vi "ATF Control Screen.vi"() -> ()   [LabVIEW 2022 SP3]
doc: "Phase III Control Screen"
uses:
  Source Code/Controls/SeCrTs-boolean ref.ctl
  Source Code/Controls/SeCrTs-EPV .ctl
  Source Code/Controls/SeCrTs-Config.ctl
  1dfbedf7-21d1-43df-8cef-e83d174d7f49.vi
  46d7290e-ac40-4aa0-9850-85fdb2ad6f4b.vi
  c4d5dcdd-4d7e-4205-ba99-f4de1c789af6.vi
  a1e086cd-08f9-4a49-a00d-64c03a58ee35.vi
  6137576e-326d-4df8-a9af-1410d5563ab4.vi
  693608e7-53a4-46b0-95d2-cfce812533db.vi
  c1522341-ff23-4fcb-8f7c-12554df804f4.vi
  26470722-db86-46b2-ac2f-fc67b99a3691.vi
  a6ca7374-ed47-4275-bc81-d54310f82728.vi
  6670e8fc-d020-4487-9323-c9679abcbb1c.vi
  a7243c24-792e-41b0-90bb-b6aaa1b4a496.vi
  95ed83e7-93bc-4bf0-ad95-9e52adbf6774.vi
  53bb0892-c25d-49a8-a007-ace4b611b4f7.vi
  288395e4-a55c-4c24-8191-a542ab318b4e.vi
  73a44b47-5b27-40e3-90b9-f1da52c45352.vi
  604e1923-8fb6-4d67-ae19-9cc1d684d709.vi
  c1583684-2215-429c-ba9c-22f0ed15bb00.vi
  4cb2d8f4-0aba-4707-8f21-22dc63107e4b.vi
  294f453b-f809-4255-8052-722f2e12d79b.vi
  79af255e-43e2-41de-a072-683097d60ae6.vi
  0f49bbc7-f368-47f6-bd6d-30b048e0a7c3.vi
  23ec587a-6275-4f9c-af37-1b729a0e349f.vi
  c5918ca7-0479-433b-be97-aa50c5bd1a7d.vi
  Source Code/UI Message handler/User Event - Stop/User Event - Stop.lvlib
  Source Code/UI Message handler/Message Queue/Message Queue.lvlib
panel:
  out "DO Health S":bool
  out "DI Health S":bool
  out "AI C Health  S":bool
  in  "Select type":enum16{"Both", "Pump", "Storage"}(ring)
  out "PXIe Error Display":string
  out "Control Screen Error Display":string
  in  "SELECT SEQUENCER FILE":string(combo)
  in  "SELECT ABORT SEQUENCE":string[](array[combo])
  out "SEQUENCE STATE":string
  in  "HOLD CDT":bool
  in  "SET":bool
  in  "T-0":timestamp
  in  "Start or Revert Sequence":bool
  in  "Get Sequence":bool
  out "COUNT DOWN TIMER":dbl format="%<%H:%M:%S%3u>t"
  out "F_EPV_1004_HSS":bool
  in  "F_EPV_1004":bool
  out "N_EPV_1091_HSS":bool
  in  "N_EPV_1091":bool
  out "F_EPV_1007_HSS":bool
  in  "F_EPV_1007":bool
  out "F_EPV_1008_HSS":bool
  in  "F_EPV_1008":bool
  out "NC_EPV_1217_HSS":bool
  in  "NC_EPV_1217":bool
  in  "NC_EPV_481":bool
  in  "NO_EPV_478R":bool
  in  "NO_EPV_477":bool
  in  "NC_EPV_56":bool
  in  "NO_EPV_122":bool
  in  "NC_EPV_61":bool
  in  "NC_EPV_1001":bool
  out "NC_EPV_481_HSS":bool
  out "NO_EPV_478R_HSS":bool
  out "NO_EPV_477_HSS":bool
  out "NC_EPV_56_HSS":bool
  out "NO_EPV_122_HSS":bool
  out "NC_EPV_61_ HSS":bool
  out "NC_EPV_1001_HSS":bool
  in  "NC_EPV_1211":bool
  in  "NO_EPV_1102":bool
  in  "NC_EPV_1214":bool
  in  "NC_EPV_1207":bool
  in  "AC_Switch":bool
  out "NC_EPV_1211_HSS":bool
  out "NO_EPV_1102_HSS":bool
  out "NC_EPV_1214_HSS":bool
  out "NC_EPV_1207_HSS":bool
  out "MS failure":bool
  out "Over current detection":bool
  out "Over power detection":bool
  out "over voltage detection":bool
  out "power failure status":bool
  out "Terminal Voltage":i32
  out "Terminal Current":i32
  out "Terminal Power":i32
  out "No .of Slaves":u8
  in  "OVP(V)":dbl format="%#_g V"
  in  "OCP(A)":dbl format="%#_g A"
  in  "OPP(W)":dbl format="%#_g W"
  in  "SET VOLTAGE":dbl format="%#_g V"
  in  "SET CURRENT":dbl format="%#_g A"
  in  "SET POWER":dbl format="%#_g W"
  in  "RT Stop":bool
  in  "DC off":bool
  in  "DC on":bool
  in  "update ppsu":bool
  in  "Ms initialize":bool
  in  "Alarm ack":bool
  in  "ABORT":bool
  in  "Connect ppsu":bool
  out "Rotational sate":string
  out "RUN ACKNOWLEDGE Atf":bool
  out "Rotational Direction":string
  out "Speed RPM":dbl format="%#_g r/min"
  out "Frequency":dbl format="%#_g Hz"
  in  "Direction ATF":bool
  out "State ATF":dbl(knob) caption="Gauge" scale=0.0..1000.0
  in  "Speed Limit 2":dbl format="%#_g S"
  in  "Speed Limit":dbl format="%#_g S"
  in  "Ki Speed":dbl format="%#_g r/m"
  in  "Kp Speed":dbl format="%#_g Hz"
  in  "Kp Current":dbl format="%#_g S"
  in  "Ki Current":dbl format="%#_g S"
  in  "Current Limit 2":dbl format="%#_g S"
  in  "Current Limit":dbl format="%#_g S"
  in  "SPEED":dbl format="%#_g r/m"
  in  "SET FREQ":dbl format="%#_g Hz"
  in  "RAMP DOWN":dbl format="%#_g S"
  in  "RAMP UP":dbl format="%#_g S"
  out "Target 2":bool
  in  "PUMP IP":string="LOCALHOST"
  out "cover":bool
  out "User":string
  out "Login screen cover":bool
  in  "Log option":cluster{"Log type":bool, "Log Period(Min)":dbl}={"Log type"=FALSE, "Log Period(Min)"=1.0}
  in  "Log In Tool":bool
  in  "Trail Number":string(combo)
  out "Log?":bool
  out "error out":errorcluster
  in  "Enable/Disable IP":bool
  out "AI C Health":bool
  out "ACC Health":bool
  out "TC Health":bool
  in  "Exit Drive ATF":bool
  out "PPSU Health":bool
  out "Target":bool
  out "Drive ATF Health":bool
  out "DO Health":bool
  out "DI Health":bool
  out "AO Health":bool
  out "AI V Health":bool
  out "Time":timestamp format="%<%.3X>T"
  in  "Datalog phase code":string(combo)
  in  "Configuration File":string(combo)="F3 test 2"
  in  "STORAGE IP":string="169.254.219.4"
  in  "ADC reset ATF":bool
  in  "MCU reset ATF":bool
  in  "Gate driver ATF":bool
  in  "Motor off ATF":bool
  in  "Motor On ATF":bool
  in  "Update drive ATF":bool
  in  "STOP LOG":bool
  in  "Connect Drive ATF":bool
  in  "HOLD UPDATE":bool
  in  "DAQ SETTING":bool
  in  "Connect RT":bool
  in  "STOP DAQ":bool
  in  "START LOG":bool
  in  "START DAQ":bool
  in  "Exit":bool
  # "ATF RIG SOFTWARE"
  # "VERSION NUMBER :4.0"
  # "RELEASE DATE : Soon...!"
  # "Select the configuration file"
  # "Select the phase code"
  # "SEQUENCE"
  # "ATF STORAGE"
  # "ATF PUMP"
  # "ATF Drive Console"
  # "PPSU CONSOLE"
  # "ATF DRIVE FEEDBACK"
  # "FEEDBACK PARAMETERS"
  # "SET PARAMETERS"
  # "FAULT STATUS"
  # "ATF DRIVE SET PARAMETERS"
  # "CW"
  # "CCW"
  # "Continuous log"
  # "Periodical log"
  # "+"
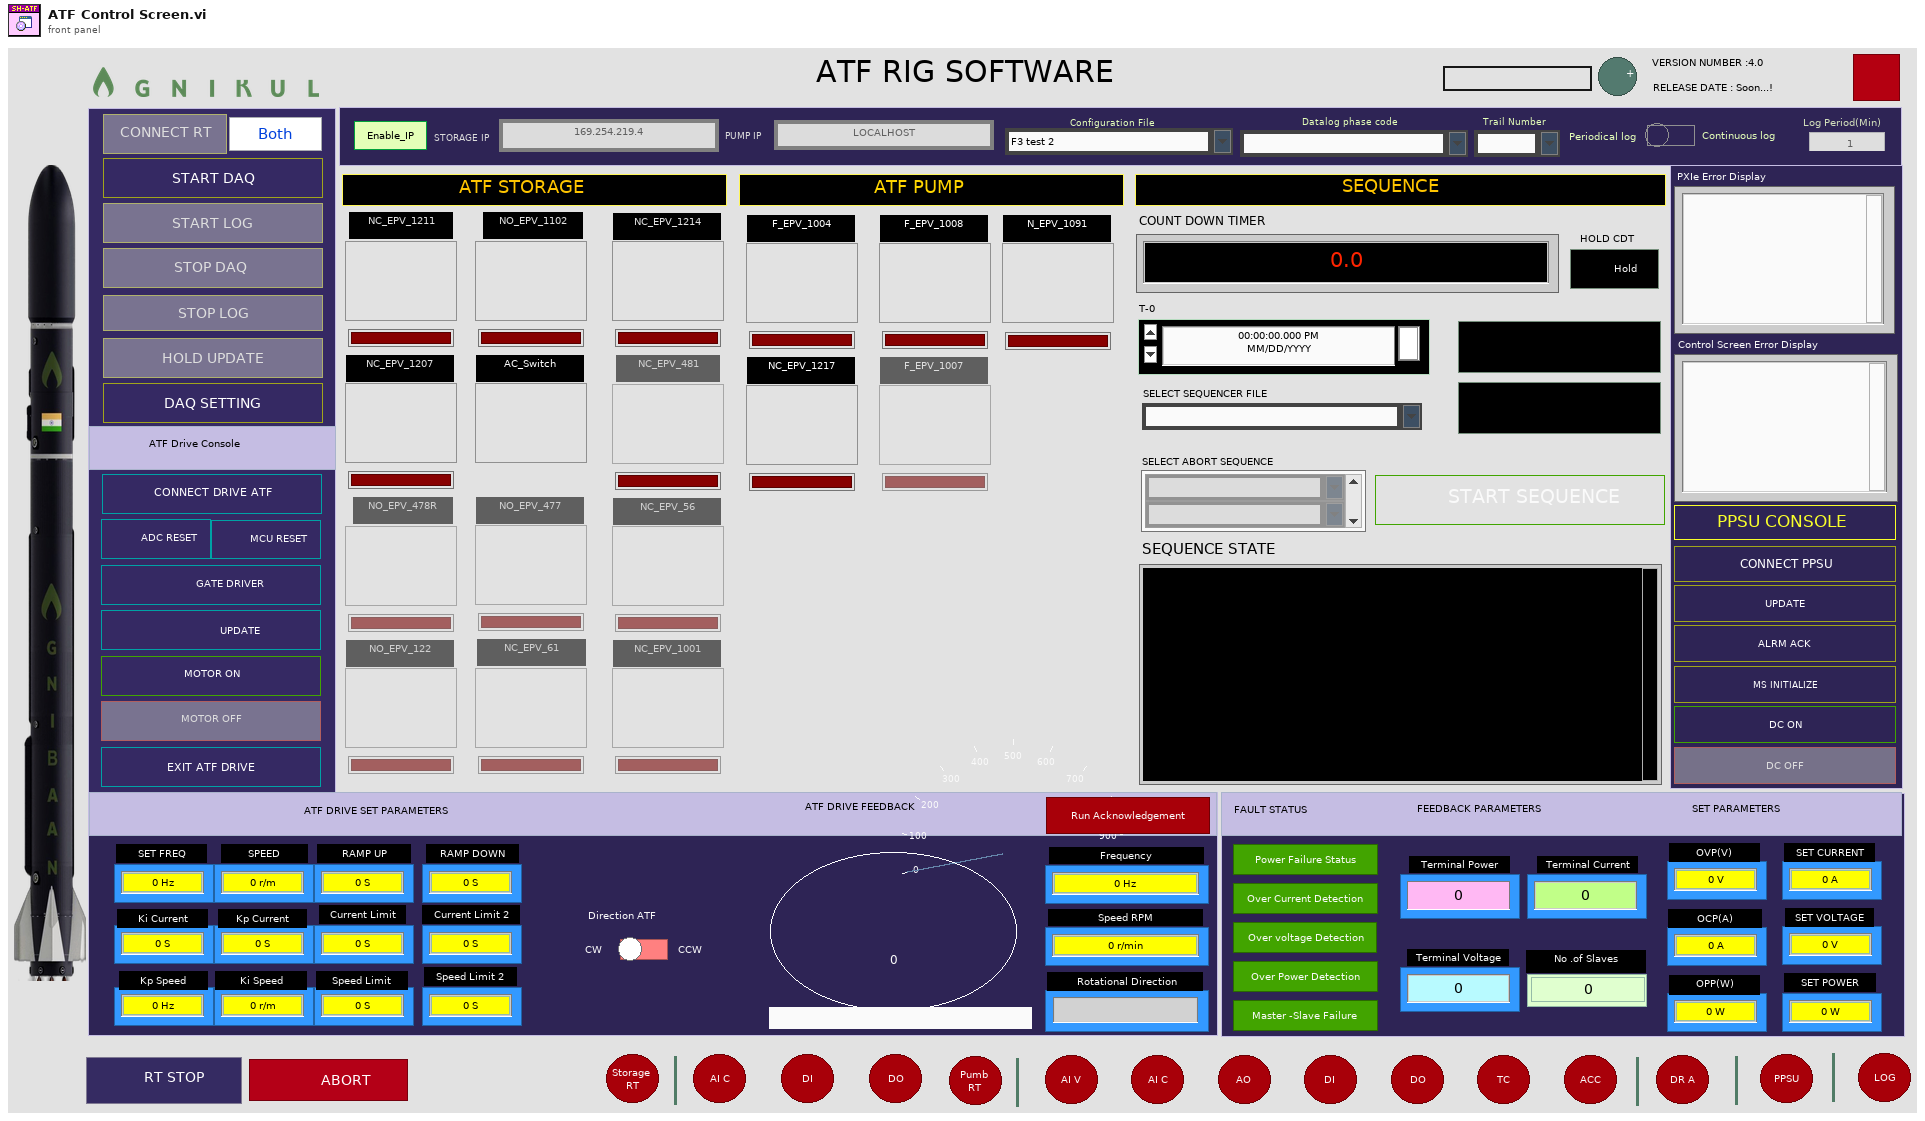
[diagram p1: front panel]
types:
  T1 = typedef "SeCrTs-boolean ref.ctl" = cluster{"Connect RT":refnum<vi>, "START DAQ":refnum<vi>, "STOP DAQ":refnum<vi>, "DAQ SETTING":refnum<vi>, "START LOG":refnum<vi>, "STOP LOG":refnum<vi>, "Connect Drive ATF":refnum<vi>, "Update drive ATF":refnum<vi>, "Gate driver ATF":refnum<vi>, "Motor On ATF":refnum<vi>, "ADC reset ATF":refnum<vi>, "Gate driver ATF 2":refnum<vi>, "Motor off ATF":refnum<vi>, "MCU reset ATF":refnum<vi>, "Connect Drive Lox":refnum<vi>, "Update drive lox":refnum<vi>, "Gate driver- LOX":refnum<vi>, "Motor On lox":refnum<vi>, "Adc reset lox":refnum<vi>, "MCU Reset -LOX":refnum<vi>, "Motor Off lox":refnum<vi>, "Connect ppsu":refnum<vi>, "update ppsu":refnum<vi>, "DC on":refnum<vi>, "Alarm ack":refnum<vi>, "DC off":refnum<vi>, "Ms initialize":refnum<vi>, "Exit RT":refnum<vi>, "ABORT":refnum<vi>, "HOLD UPDATE":refnum<vi>, "Log type":refnum<vi>}
  T2 = typedef "SeCrTs-EPV .ctl" = cluster{"F_EPV_131":refnum<vi>, "F_EPV_132":refnum<vi>, "F_EPV_136":refnum<vi>, "F_EPV_21":refnum<vi>, "F_EPV_41":refnum<vi>, "N_EPV_68":refnum<vi>, "N_EPV_ 69":refnum<vi>, "N_EPV_ 33":refnum<vi>, "F_EPV_142":refnum<vi>, "F_EPV_28":refnum<vi>, "N_EPV_203":refnum<vi>, "N_EPV_206":refnum<vi>, "F_EPV_75":refnum<vi>, "C_EPV_2":refnum<vi>, "C_EPV_7":refnum<vi>, "C_EPV_8":refnum<vi>, "C_EPV_123":refnum<vi>, "C_EPV_124":refnum<vi>, "C_EPV_127":refnum<vi>, "N_EPV_62a":refnum<vi>, "N_EPV_62b":refnum<vi>, "N_EPV_61":refnum<vi>, "G_EPV_51":refnum<vi>, "N_EPV_141":refnum<vi>, "C_EPV_803":refnum<vi>, "C_EPV_18":refnum<vi>, "C_EPV_1352":refnum<vi>, "N_EPV_202":refnum<vi>, "C_EPV_16":refnum<vi>}
  T3 = cluster{"Bol":T1, "EPV":T2, "Covers":cluster{"cover":refnum<vi>, "Login screen cover":refnum<vi>, "cover Motor":refnum<vi>}, "Log cmd":cluster{"C/NC":bool, "Start/Stop Log":bool[], "Log Name":string, "Config":cluster{"AO config":cluster{"Channel_Name":string, "Channel_Number":string, "Default_Value":dbl, "Units":string}[], "AI config":cluster{"Channel_Name":string, "Channel_Number":string, "Pre_Scale_min":dbl, "Pre_Scale_max":dbl, "Sensor_min":dbl, "Sensor_max":dbl, "Units":string}[], "DI config":cluster{"Channel_Name":string, "Channel_Number":string, "Default_Value":bool, "DI invert?":bool}[], "DO config":cluster{"Channel_Name":string, "Channel_Number":string, "Default_Value":bool, "DO invert?":bool}[], "TC config":cluster{"Channel_Name":string, "Channel_Number":string, "Pre_Scale_min":dbl, "Pre_Scale_max":dbl, "units":i32, " type":i32}[], "ACC config":cluster{"Channel_Name":string, "Channel_Number":string, "Pre_Scale_min":dbl, "Pre_Scale_max":dbl, "Terminal configuration":i32, "Sensitivity":dbl, "Sensitivity units":i32}[], "SG config":cluster{"Channel_Name":string, "Channel_Number":string, "Pre_Scale_min":dbl, "Pre_Scale_max":dbl}[], "Strain Gauge Settings":cluster{"poisson ratio":dbl, "nominal gage resistance":dbl, "gage factor":dbl}, "Bridge Settings":cluster{"voltage excitation value":dbl, "voltage excitation source":i32, "initial bridge voltage":dbl, "lead wire resistance":dbl, "strain configuration":i32}, "Sample Rate":cluster{"AI Sample Rate":dbl[], "AO Sample Rate":dbl[], "DI Sample Rate":dbl[], "TC Sample Rate":dbl[], "DO Sample Rate":dbl[], "SG Sample Rate":dbl[], "ACC Sample Rate":dbl[]}}, "Log min":dbl}}
  T4 = enum16{"Init", "Read 'All'", "Read 'n'", "Read '1'", "Write '1'", "Write 'n'", "Write 'All'"}
  T5 = typedef "SeCrTs-Notifier ctl.ctl" = cluster{"Storage Data":refnum<notifier>, "Pumb Data":refnum<notifier>, "Log cmd":refnum<notifier>}
  T6 = typedef "Message Queue.lvlib/All Message Queues.ctl" = cluster{"UI":refnum<queue>, "ER":refnum<queue>, "Ev":refnum<queue>, "R ER Storage":refnum<queue>, "PPSU":refnum<queue>, "R ER Pumb":refnum<queue>}
  T7 = enum8{"Enabled", "Disabled", "Disabled and Grayed Out"}
  T8 = typedef "SeCrTs-Config.ctl" = cluster{"AO config":cluster{"Channel_Name":string, "Channel_Number":string, "Default_Value":dbl, "Units":string}[], "AI config":cluster{"Channel_Name":string, "Channel_Number":string, "Pre_Scale_min":dbl, "Pre_Scale_max":dbl, "Sensor_min":dbl, "Sensor_max":dbl, "Units":string}[], "DI config":cluster{"Channel_Name":string, "Channel_Number":string, "Default_Value":bool, "DI invert?":bool}[], "DO config":cluster{"Channel_Name":string, "Channel_Number":string, "Default_Value":bool, "DO invert?":bool}[], "TC config":cluster{"Channel_Name":string, "Channel_Number":string, "Pre_Scale_min":dbl, "Pre_Scale_max":dbl, "units":i32, " type":i32}[], "ACC config":cluster{"Channel_Name":string, "Channel_Number":string, "Pre_Scale_min":dbl, "Pre_Scale_max":dbl, "Terminal configuration":i32, "Sensitivity":dbl, "Sensitivity units":i32}[], "SG config":cluster{"Channel_Name":string, "Channel_Number":string, "Pre_Scale_min":dbl, "Pre_Scale_max":dbl}[], "Strain Gauge Settings":cluster{"poisson ratio":dbl, "nominal gage resistance":dbl, "gage factor":dbl}, "Bridge Settings":cluster{"voltage excitation value":dbl, "voltage excitation source":i32, "initial bridge voltage":dbl, "lead wire resistance":dbl, "strain configuration":i32}, "Sample Rate":cluster{"AI Sample Rate":dbl[], "AO Sample Rate":dbl[], "DI Sample Rate":dbl[], "TC Sample Rate":dbl[], "DO Sample Rate":dbl[], "SG Sample Rate":dbl[], "ACC Sample Rate":dbl[]}}
  T9 = enum16{"open", "replace", "create", "open or create", "replace or create", "replace or create with confirmation"}
  T10 = cluster{"OPP(W)":dbl, "OVP(V)":dbl, "OCP(A)":dbl, "SET VOLTAGE":dbl, "SET CURRENT":dbl, "SET POWER":dbl}
  T11 = typedef "SeCrTs-file folder ctl.ctl" = cluster{"Datalog path":path, "Configuration path":path, "Signal list path":path, "Sub vi's":path, "Authentication":path, "Sequence":path, "Event Log":path, "CS Error log":path, "RT Error Log":path}
  T12 = enum8{"Enabled", "Disabled", "Disabled and Grayed Out"}[]
  T13 = cluster{"cover":refnum<vi>, "Login screen cover":refnum<vi>, "cover Motor":refnum<vi>}
  T14 = cluster{"C/NC":bool, "Start/Stop Log":bool[], "Log Name":string, "Config":cluster{"AO config":cluster{"Channel_Name":string, "Channel_Number":string, "Default_Value":dbl, "Units":string}[], "AI config":cluster{"Channel_Name":string, "Channel_Number":string, "Pre_Scale_min":dbl, "Pre_Scale_max":dbl, "Sensor_min":dbl, "Sensor_max":dbl, "Units":string}[], "DI config":cluster{"Channel_Name":string, "Channel_Number":string, "Default_Value":bool, "DI invert?":bool}[], "DO config":cluster{"Channel_Name":string, "Channel_Number":string, "Default_Value":bool, "DO invert?":bool}[], "TC config":cluster{"Channel_Name":string, "Channel_Number":string, "Pre_Scale_min":dbl, "Pre_Scale_max":dbl, "units":i32, " type":i32}[], "ACC config":cluster{"Channel_Name":string, "Channel_Number":string, "Pre_Scale_min":dbl, "Pre_Scale_max":dbl, "Terminal configuration":i32, "Sensitivity":dbl, "Sensitivity units":i32}[], "SG config":cluster{"Channel_Name":string, "Channel_Number":string, "Pre_Scale_min":dbl, "Pre_Scale_max":dbl}[], "Strain Gauge Settings":cluster{"poisson ratio":dbl, "nominal gage resistance":dbl, "gage factor":dbl}, "Bridge Settings":cluster{"voltage excitation value":dbl, "voltage excitation source":i32, "initial bridge voltage":dbl, "lead wire resistance":dbl, "strain configuration":i32}, "Sample Rate":cluster{"AI Sample Rate":dbl[], "AO Sample Rate":dbl[], "DI Sample Rate":dbl[], "TC Sample Rate":dbl[], "DO Sample Rate":dbl[], "SG Sample Rate":dbl[], "ACC Sample Rate":dbl[]}}, "Log min":dbl}
  T15 = cluster{cluster{"Sr. No.":string, "Time CDT":string, "Component ID":string, "Data Type":string, "Condition":string, "Range/Position":string, "No of Samples for Pass":string, "Event Duration":string, "Continuous /Cumulative":string, "Expected Delay":string, "Failure case Seq":string, "Current Sequence":string}[]}[]
  T16 = cluster{"Sr. No.":string, "Time CDT":string, "Component ID":string, "Data Type":string, "Condition":string, "Range/Position":string, "No of Samples for Pass":string, "Event Duration":string, "Continuous /Cumulative":string, "Expected Delay":string, "Failure case Seq":string, "Current Sequence":string}[]
  T17 = cluster{"[0]":dbl, "[1]":dbl, "[2]":dbl, "[3]":dbl, "[4]":dbl, "[5]":dbl, "[6]":dbl, "[7]":dbl, "[8]":dbl}
  T18 = cluster{"Error Code":string, "Error Source":string}
  T19 = typedef "SeCrTs-NS Data type.ctl" = cluster{"DI_Data":digitalwaveform[], "Drive_A_C":waveform(dbl)[], "Drive_A_D":waveform(dbl)[], "Drive_L_C":waveform(dbl)[], "Drive_L_D":waveform(dbl)[], "Loop Status":bool[], "CDT":dbl, "RT Error":cluster{"Error Code":string, "Error Source":string}, "DO":waveform(dbl)[], "SEQ Monitor":string[], "Device List":string}
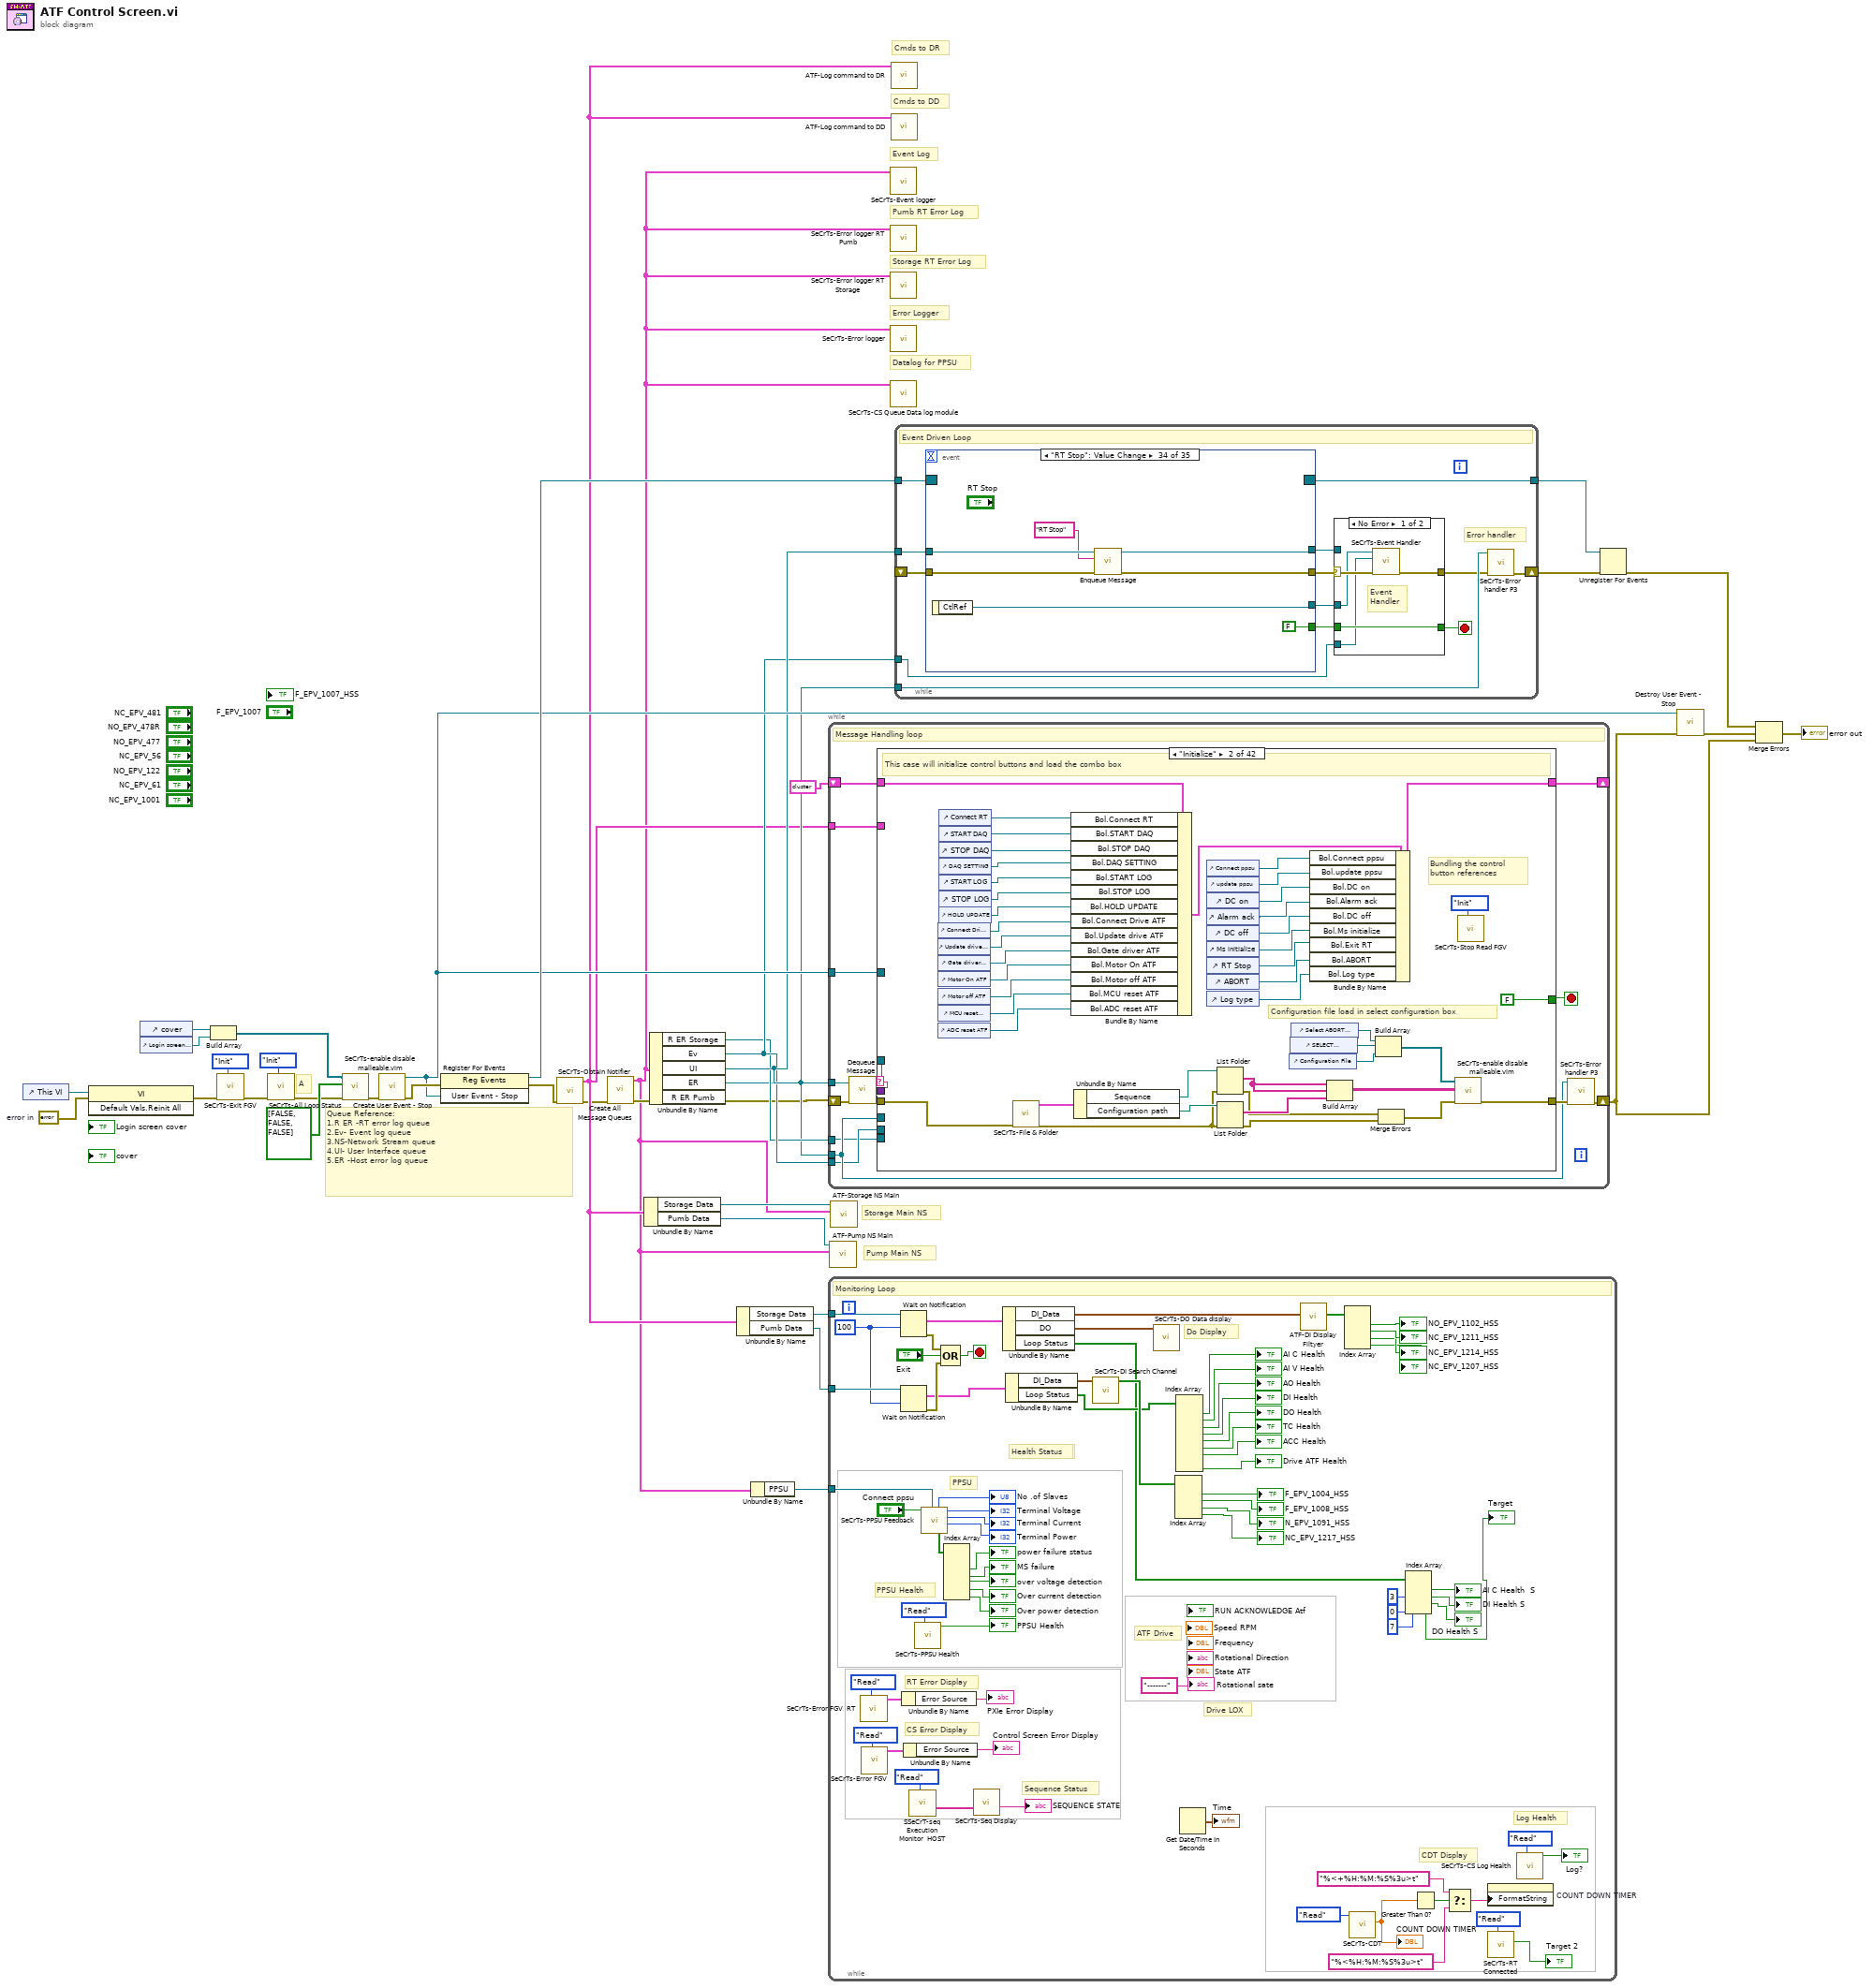
[diagram p0: block diagram]
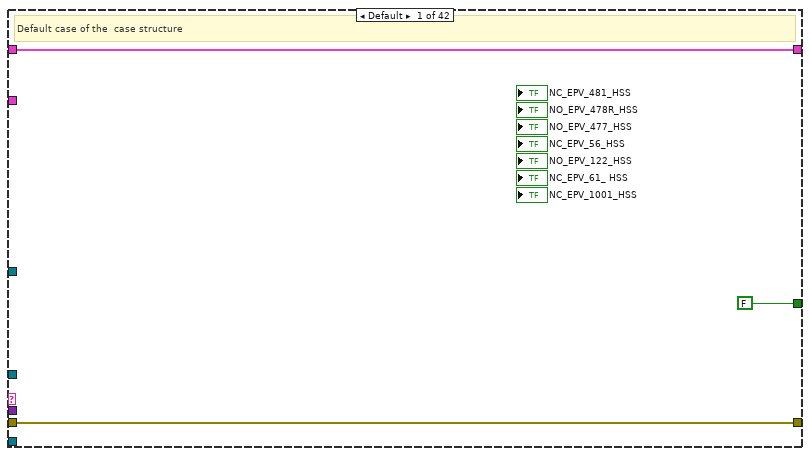
[diagram p2: hidden frame]
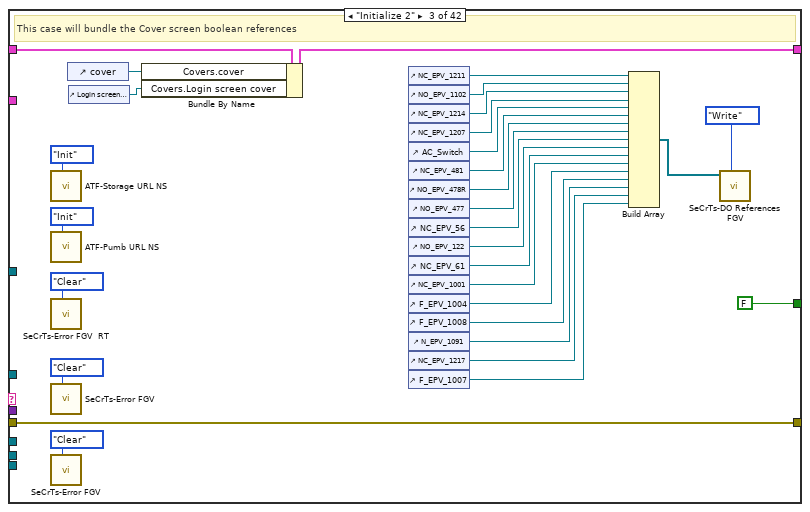
[diagram p3: hidden frame]
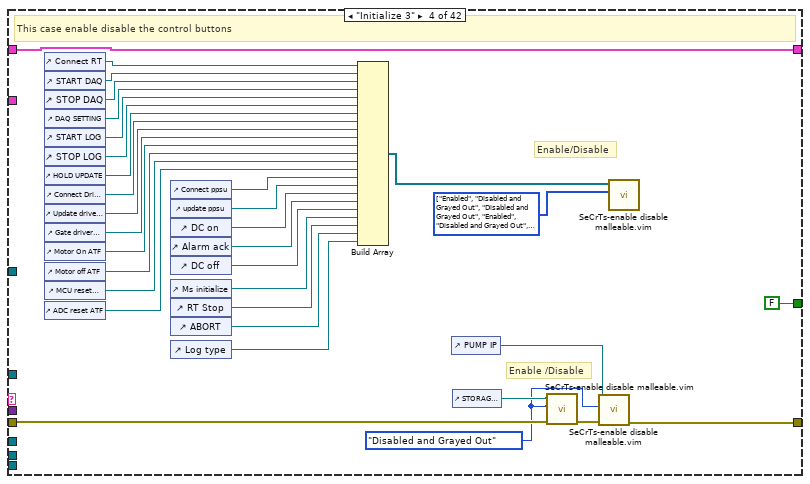
[diagram p4: hidden frame]
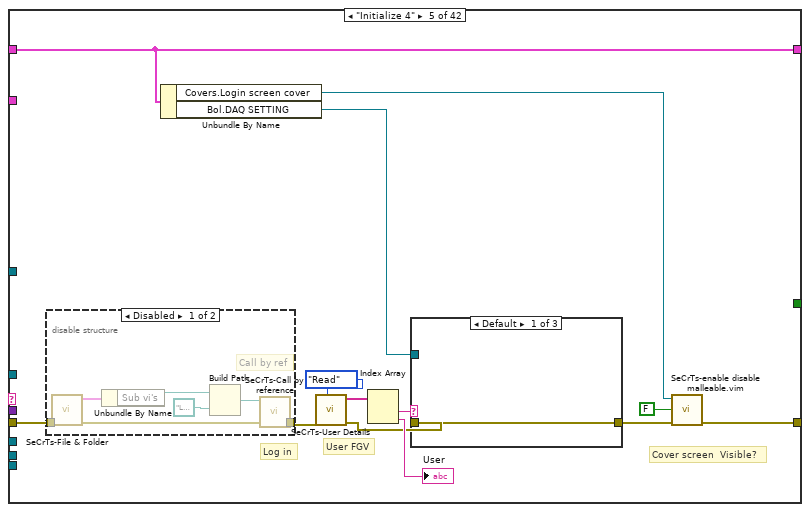
[diagram p5: hidden frame]
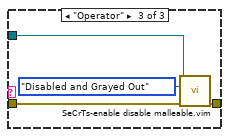
[diagram p8: hidden frame]
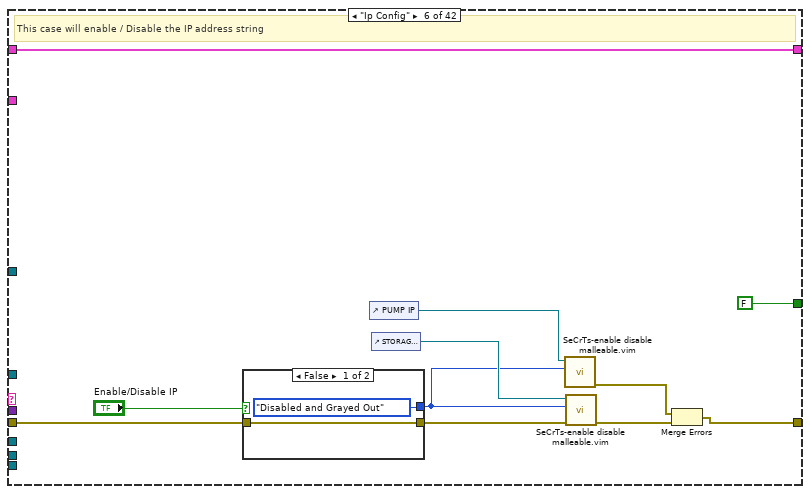
[diagram p9: hidden frame]
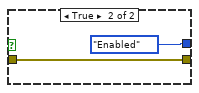
[diagram p10: hidden frame]
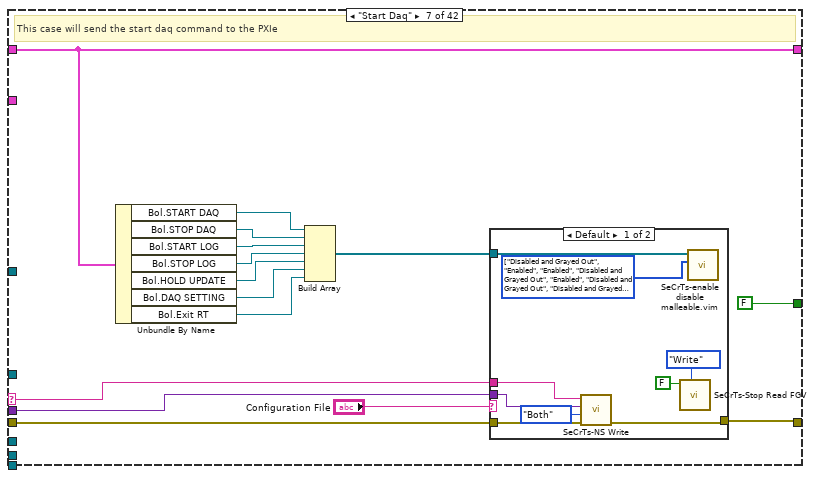
[diagram p11: hidden frame]
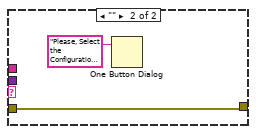
[diagram p12: hidden frame]
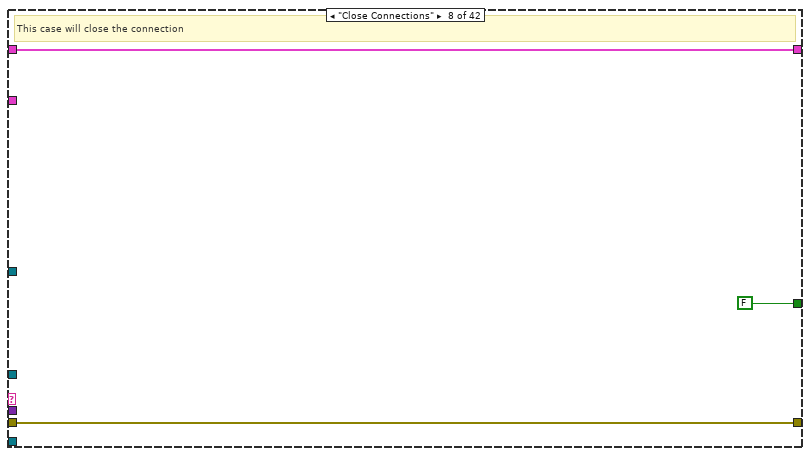
[diagram p13: hidden frame]
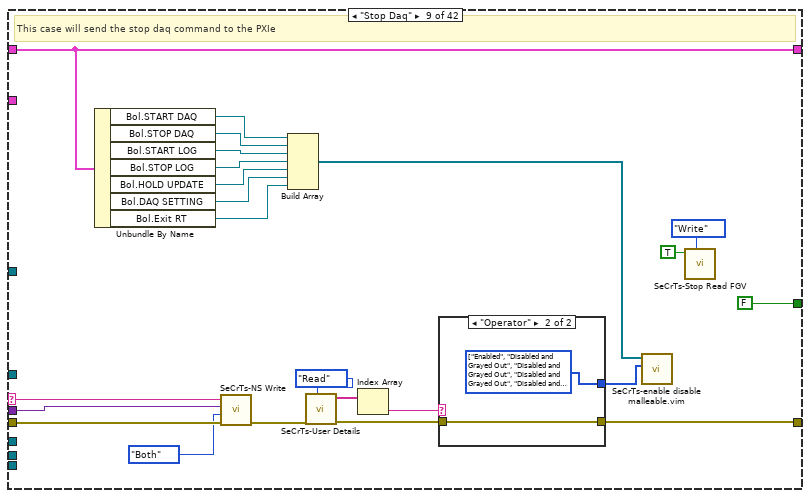
[diagram p14: hidden frame]
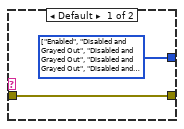
[diagram p15: hidden frame]
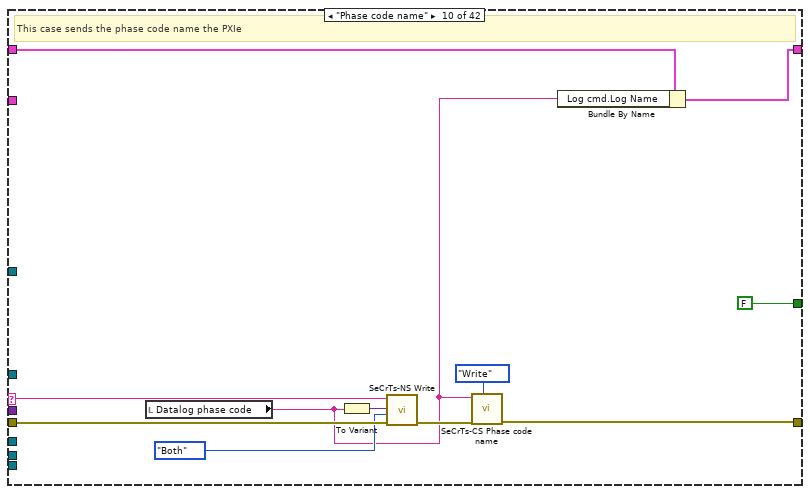
[diagram p16: hidden frame]
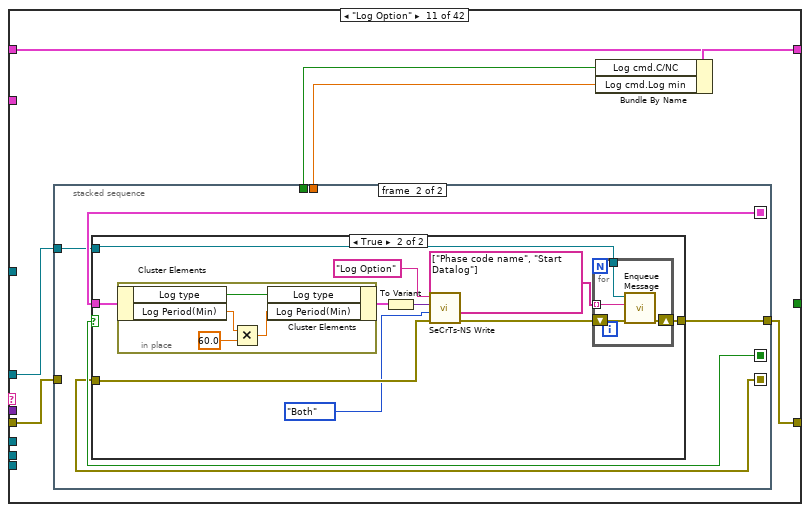
[diagram p17: hidden frame]
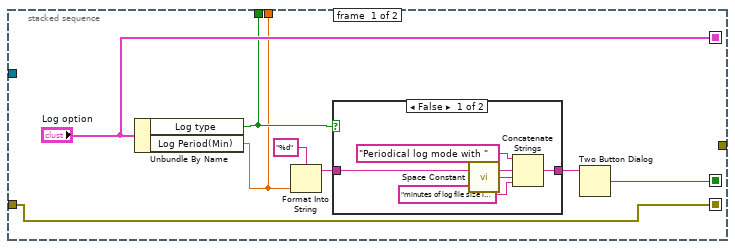
[diagram p18: hidden frame]
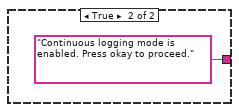
[diagram p19: hidden frame]
diagram:
  w27 = errorcluster {"status"=FALSE, "code"=0, "source"=""}  # error in
  # "Cmds to DD"
  # "Cmds to DR"
  # "Pump Main NS"
  # "Pumb RT Error Log"
  # "A"
  # "Queue Reference:\n1.R ER -RT error log queue\n2.Ev- Event log queue\n3.NS-Network Stream queue\n4.UI- User Interface queue\n5.ER -Host error log queue"
  # "Event Log"
  # "Storage Main NS"
  # "Storage RT Error Log"
  # "Error Logger"
  # "Datalog for PPSU"
  n1 = control-ref of="This VI"() -> (w28:refnum<vi>)
  n2 = invoke on="Invoke Node" class="VI" method="Default Vals.Reinit All"(reference=w28, error in=w27) -> (error out=w12:errorcluster)  [unwired: 1 in, 2 out]
  n3 = control-ref of="cover"() -> (w23:refnum<vi>)
  n4 = control-ref of="Login screen cover"() -> (w22:refnum<vi>)
  n5 = Build Array(w23, w22) -> (w10:refnum<vi>[])
  n6 = call "SeCrTs-Exit FGV.vi"("Enum"=enum16{"Init", "Read", "Write"}."Init", "error in"=w12) -> ("error out"=w11:errorcluster)  [unwired: 8 in, 1 out]
  n7 = call "SeCrTs-All Loop Status.vi"("Option"=T4."Init", "error in (no error)"=w11) -> ("error out"=w8:errorcluster)  [unwired: 7 in, 2 out]
  n8 = call "SeCrTs-enable disable malleable.vim"("error in"=w8, "Data"=bool[] [FALSE, FALSE, FALSE] ("Visible"), "Ref in"=w10) -> ("error out"=w7:errorcluster)  [unwired: 8 in]
  n9 = call "Create User Event - Stop.vi"("error in (no error)"=w7) -> ("error out"=w33:errorcluster, "User Event - Stop"=w24:refnum<user-event>)  [unwired: 9 in]
  n10 = register-events(error in=w33, w24) -> (reference out=w36:refnum<event-registration>, error out=w30:errorcluster)  [unwired: 1 in]
  n11 = call "SeCrTs-Obtain Notifier.vi"("error in"=w30) -> ("error out"=w1:errorcluster, "Cluster"=w4:T5)  [unwired: 9 in]
  n12 = call "Create All Message Queues.vi"("error in (no error)"=w1) -> ("error out"=w6:errorcluster, "Message Queues out"=w3:T6)  [unwired: 9 in]
  n13 = Unbundle By Name(w4) -> ("Storage Data"=w14:refnum<notifier>, "Pumb Data"=w2:refnum<notifier>)
  n14 = Unbundle By Name(w3) -> ("R ER Storage"=w16:refnum<queue>, "Ev"=w17:refnum<queue>, "UI"=w18:refnum<queue>, "ER"=w13:refnum<queue>)  [unwired: 1 out]
  n15 = Unbundle By Name(w4) -> ("Storage Data"=w29:refnum<notifier>, "Pumb Data"=w5:refnum<notifier>)
  n16 = Unbundle By Name(w3) -> ("PPSU"=w15:refnum<queue>)
  n17 = while {
    shift-right: [w40] -> w19
    shift-left: w6 -> [w50]
    tunnel: w24 -> [w51]
    tunnel: w18 -> [w44]
    tunnel: w4 -> [w45]
    shift-right: [w42] -> _
    shift-left: T3 {"Bol"={"Connect RT"=refnum, "START DAQ"=refnum, "STOP DAQ"=refnum, "DAQ SETTING"=refnum, "START LOG"=refnum, "STOP LOG"=refnum, "Connect Drive ATF"=refnum, "Update drive ATF"=refnum, "Gate driver ATF"=refnum, "Motor On ATF"=refnum, "ADC reset ATF"=refnum, "Gate driver ATF 2"=refnum, "Motor off ATF"=refnum, "MCU reset ATF"=refnum, "Connect Drive Lox"=refnum, "Update drive lox"=refnum, "Gate driver- LOX"=refnum, "Motor On lox"=refnum, "Adc reset lox"=refnum, "MCU Reset -LOX"=refnum, "Motor Off lox"=refnum, "Connect ppsu"=refnum, "update ppsu"=refnum, "DC on"=refnum, "Alarm ack"=refnum, "DC off"=refnum, "Ms initialize"=refnum, "Exit RT"=refnum, "ABORT"=refnum, "HOLD UPDATE"=refnum, "Log type"=refnum}, "EPV"={"F_EPV_131"=refnum, "F_EPV_132"=refnum, "F_EPV_136"=refnum, "F_EPV_21"=refnum, "F_EPV_41"=refnum, "N_EPV_68"=refnum, "N_EPV_ 69"=refnum, "N_EPV_ 33"=refnum, "F_EPV_142"=refnum, "F_EPV_28"=refnum, "N_EPV_203"=refnum, "N_EPV_206"=refnum, "F_EPV_75"=refnum, "C_EPV_2"=refnum, "C_EPV_7"=refnum, "C_EPV_8"=refnum, "C_EPV_123"=refnum, "C_EPV_124"=refnum, "C_EPV_127"=refnum, "N_EPV_62a"=refnum, "N_EPV_62b"=refnum, "N_EPV_61"=refnum, "G_EPV_51"=refnum, "N_EPV_141"=refnum, "C_EPV_803"=refnum, "C_EPV_18"=refnum, "C_EPV_1352"=refnum, "N_EPV_202"=refnum, "C_EPV_16"=refnum}, "Covers"={"cover"=refnum, "Login screen cover"=refnum, "cover Motor"=refnum}, "Log cmd"={"C/NC"=FALSE, "Start/Stop Log"=[], "Log Name"="", "Config"={"AO config"=[], "AI config"=[], "DI config"=[], "DO config"=[], "TC config"=[], "ACC config"=[], "SG config"=[], "Strain Gauge Settings"={"poisson ratio"=0.0, "nominal gage resistance"=0.0, "gage factor"=0.0}, "Bridge Settings"={"voltage excitation value"=0.0, "voltage excitation source"=0, "initial bridge voltage"=0.0, "lead wire resistance"=0.0, "strain configuration"=0}, "Sample Rate"={"AI Sample Rate"=[], "AO Sample Rate"=[], "DI Sample Rate"=[], "TC Sample Rate"=[], "DO Sample Rate"=[], "SG Sample Rate"=[], "ACC Sample Rate"=[]}}, "Log min"=0.0}} -> [w43]
    tunnel: w13 -> [w39]
    tunnel: w17 -> [w38]
    tunnel: w16 -> [w37]
    stop <- w52 stop-if-true
    # "Message Handling loop"
    n18 = call "Dequeue Message.vi"("error in (no error)"=w50, "Message Queue"=w44) -> ("error out"=w49:errorcluster, "Message Data"=w46:variant, "Message"=w48:string, "dup Message Queue"=w47:refnum<queue>)  [unwired: 6 in]
    n19 = case shown="\"Initialize\"" w48 {
      selector: w48 -> [_ _ _ _ _ _ w217 _ w254 w269 _ _ _ _ _ _ _ _ _ _ _ _ w564 _ w592 _ _ _ _ _ _ _ _ _ _ w687 _ w715 w726 _ _ _]
      tunnel: w49 -> [w55 w73 w122 w136 w172 w197 w205 w232 w253 w270 w277 w340 w367 w392 w404 _ w454 w460 w496 w524 w538 w560 w566 w572 w593 w598 w601 w603 w617 w632 w639 w648 w660 w674 w678 w686 w690 w717 w728 w745 w748 w750]
      tunnel: [w55 w59 w122 w132 w165 w193 w216 w232 w238 w264 w275 w331 w371 w391 w399 w424 w452 w457 w493 w504 w535 w559 w563 w570 w590 w598 w601 w602 w616 w631 w638 w647 w658 w673 w677 w688 w693 w703 w727 w736 w748 w749] -> w41
      tunnel: [FALSE ("EXIT") FALSE ("EXIT") FALSE ("EXIT") FALSE ("EXIT") _ FALSE ("EXIT") FALSE ("EXIT") FALSE ("EXIT") FALSE ("EXIT") FALSE ("EXIT") _ FALSE ("EXIT") FALSE ("EXIT") FALSE ("EXIT") FALSE ("EXIT") FALSE ("EXIT") FALSE ("EXIT") FALSE ("EXIT") FALSE ("EXIT") FALSE ("EXIT") FALSE ("EXIT") FALSE ("EXIT") FALSE ("EXIT") FALSE ("EXIT") FALSE ("EXIT") FALSE ("EXIT") FALSE ("EXIT") FALSE ("EXIT") FALSE ("EXIT") FALSE ("EXIT") FALSE ("EXIT") FALSE ("EXIT") FALSE ("EXIT") FALSE ("EXIT") FALSE ("EXIT") FALSE ("EXIT") FALSE ("EXIT") TRUE ("EXIT") FALSE ("EXIT") FALSE ("EXIT") FALSE ("EXIT") FALSE ("EXIT")] -> w52
      tunnel: w51 -> [_ _ _ _ _ _ _ _ _ _ _ _ _ _ _ _ _ _ _ _ _ _ _ _ _ _ _ _ _ _ _ _ _ _ _ _ _ w714 _ _ _ _]
      tunnel: w47 -> [_ _ _ _ _ _ _ _ _ _ w276 _ _ _ _ _ _ _ _ _ _ _ _ _ _ _ _ _ _ _ _ _ _ _ _ _ _ _ _ _ _ _]
      tunnel: w46 -> [_ _ _ _ _ _ w218 _ w255 _ _ _ _ _ _ _ _ _ _ _ _ _ _ _ w591 _ _ _ _ _ _ _ _ _ _ _ _ _ _ _ _ _]
      tunnel: w45 -> [_ _ _ _ _ _ _ _ _ _ _ w325 w365 _ _ _ _ _ _ _ _ _ _ _ _ _ _ _ _ _ _ _ _ _ _ _ _ w719 _ _ _ _]
      tunnel: w43 -> [w54 w66 w128 w139 w171 w199 w207 w231 w245 w261 w273 w322 w360 w389 w394 w443 w455 w472 w491 w505 w542 w561 w569 w574 w595 w597 w600 w608 w623 w633 w637 w650 w657 w676 w680 w682 w691 w713 w722 w732 w747 w757]
      tunnel: [w54 w65 w127 w139 w171 w199 w207 w231 w245 w262 w274 w323 w361 w389 w395 w443 w455 w472 w491 w505 w542 w561 w569 w574 w595 w597 w600 w608 w623 w633 w637 w650 w657 w676 w680 w682 w691 w713 w722 w732 w747 w757] -> w42
      tunnel: w39 -> [_ _ _ _ _ _ _ _ _ _ _ _ _ _ _ _ _ _ _ _ _ _ _ _ _ _ _ _ _ _ _ _ _ _ _ _ _ w708 _ _ _ _]
      tunnel: w38 -> [_ _ _ _ _ _ _ _ _ _ _ _ _ _ _ _ _ _ _ _ _ _ _ _ _ _ _ _ _ _ _ _ _ _ _ _ _ w706 _ _ _ _]
      tunnel: w37 -> [_ _ _ _ _ _ _ _ _ _ _ _ _ _ _ _ _ _ _ _ _ _ _ _ _ _ _ _ _ _ _ _ _ _ _ _ _ w704 _ _ _ _]
      frame Default {
        # "Default case of the  case structure"
      }
      frame "Initialize" {
        # "Configuration file load in select configuration box"
        # "Bundling the control \nbutton references"
        # "This case will initialize control buttons and load the combo box"
        n20 = control-ref of="Connect Drive ATF"() -> (w92:refnum<vi>)
        n21 = control-ref of="Update drive ATF"() -> (w91:refnum<vi>)
        n22 = control-ref of="Gate driver ATF"() -> (w90:refnum<vi>)
        n23 = control-ref of="Motor On ATF"() -> (w89:refnum<vi>)
        n24 = control-ref of="Motor off ATF"() -> (w88:refnum<vi>)
        n25 = control-ref of="MCU reset ATF"() -> (w87:refnum<vi>)
        n26 = control-ref of="ADC reset ATF"() -> (w86:refnum<vi>)
        n27 = control-ref of="Connect RT"() -> (w99:refnum<vi>)
        n28 = control-ref of="START DAQ"() -> (w98:refnum<vi>)
        n29 = control-ref of="STOP DAQ"() -> (w97:refnum<vi>)
        n30 = control-ref of="DAQ SETTING"() -> (w96:refnum<vi>)
        n31 = control-ref of="START LOG"() -> (w95:refnum<vi>)
        n32 = control-ref of="STOP LOG"() -> (w94:refnum<vi>)
        n33 = control-ref of="HOLD UPDATE"() -> (w93:refnum<vi>)
        n34 = call "SeCrTs-File & Folder.vi"("error in (no error)"=w73) -> ("error out"=w71:errorcluster, "File Output"=w74:T11)  [unwired: 9 in]
        n35 = Bundle By Name(cluster=w66, "Bol.Connect RT"=w99, "Bol.START DAQ"=w98, "Bol.STOP DAQ"=w97, "Bol.DAQ SETTING"=w96, "Bol.START LOG"=w95, "Bol.STOP LOG"=w94, "Bol.HOLD UPDATE"=w93, "Bol.Connect Drive ATF"=w92, "Bol.Update drive ATF"=w91, "Bol.Gate driver ATF"=w90, "Bol.Motor On ATF"=w89, "Bol.Motor off ATF"=w88, "Bol.MCU reset ATF"=w87, "Bol.ADC reset ATF"=w86) -> (w85:T3)
        n36 = Unbundle By Name(w74) -> ("Sequence"=w72:path, "Configuration path"=w75:path)
        n37 = control-ref of="Connect ppsu"() -> (w84:refnum<vi>)
        n38 = control-ref of="update ppsu"() -> (w83:refnum<vi>)
        n39 = control-ref of="DC on"() -> (w82:refnum<vi>)
        n40 = control-ref of="Alarm ack"() -> (w81:refnum<vi>)
        n41 = control-ref of="DC off"() -> (w80:refnum<vi>)
        n42 = control-ref of="Ms initialize"() -> (w79:refnum<vi>)
        n43 = control-ref of="RT Stop"() -> (w78:refnum<vi>)
        n44 = control-ref of="ABORT"() -> (w77:refnum<vi>)
        n45 = control-ref of="Log type"() -> (w60:refnum<vi>)
        n46 = List Folder(path=w72, error in=w71) -> (filenames=w63:string[], error out=w69:errorcluster)  [unwired: 2 in, 2 out]
        n47 = List Folder(path=w75, error in=w71) -> (filenames=w70:string[], error out=w76:errorcluster)  [unwired: 2 in, 2 out]
        n48 = control-ref of="Configuration File"() -> (w68:refnum<vi>)
        n49 = control-ref of="SELECT SEQUENCER FILE"() -> (w67:refnum<vi>)
        n50 = control-ref of="Select ABORT SEQUENCE"() -> (w62:refnum<vi>)
        n51 = Bundle By Name(cluster=w85, "Bol.Connect ppsu"=w84, "Bol.update ppsu"=w83, "Bol.DC on"=w82, "Bol.Alarm ack"=w81, "Bol.DC off"=w80, "Bol.Ms initialize"=w79, "Bol.Exit RT"=w78, "Bol.ABORT"=w77, "Bol.Log type"=w60) -> (w65:T3)
        n52 = Build Array(w63, w63, w70) -> (w56:string[][])
        n53 = Build Array(w62, w67, w68) -> (w57:refnum<vi>[])
        n54 = Merge Errors(w69, w76) -> (w58:errorcluster)
        n55 = call "SeCrTs-enable disable malleable.vim"("error in"=w58, "Data"=w56, "Ref in"=w57) -> ("error out"=w59:errorcluster)  [unwired: 8 in]
        n56 = call "SeCrTs-Stop Read FGV.vi"("Enum"=enum16{"Init", "Read", "Write"}."Init") -> ()  [unwired: 10 in, 1 out]
      }
      frame "Initialize 2" {
        # "This case will bundle the Cover screen boolean references"
        n57 = call "ATF-Storage URL NS.vi"("Enum"=enum16{"Init", "Read", "Write"}."Init") -> ()  [unwired: 9 in, 2 out]
        n58 = call "ATF-Pumb URL NS.vi"("Enum"=enum16{"Init", "Read", "Write"}."Init") -> ()  [unwired: 9 in, 2 out]
        n59 = call "SeCrTs-Error FGV  RT.vi"("Enum"=enum16{"Read", "Write", "Clear"}."Clear") -> ()  [unwired: 10 in, 1 out]
        n60 = call "SeCrTs-Error FGV.vi"("Enum"=enum16{"Read", "Write", "Clear"}."Clear") -> ()  [unwired: 10 in, 1 out]
        n61 = call "SeCrTs-Error FGV.vi"("Enum"=enum16{"Read", "Write", "Clear"}."Clear") -> ()  [unwired: 10 in, 1 out]
        n62 = control-ref of="cover"() -> (w126:refnum<vi>)
        n63 = control-ref of="Login screen cover"() -> (w125:refnum<vi>)
        n64 = Bundle By Name(cluster=w128, "Covers.cover"=w126, "Covers.Login screen cover"=w125) -> (w127:T3)
        n65 = control-ref of="NC_EPV_1211"() -> (w101:refnum<vi>)
        n66 = control-ref of="NO_EPV_1102"() -> (w102:refnum<vi>)
        n67 = control-ref of="NC_EPV_1214"() -> (w103:refnum<vi>)
        n68 = control-ref of="NC_EPV_1207"() -> (w104:refnum<vi>)
        n69 = control-ref of="AC_Switch"() -> (w105:refnum<vi>)
        n70 = control-ref of="NC_EPV_481"() -> (w106:refnum<vi>)
        n71 = control-ref of="NO_EPV_478R"() -> (w107:refnum<vi>)
        n72 = control-ref of="NO_EPV_477"() -> (w108:refnum<vi>)
        n73 = control-ref of="NC_EPV_56"() -> (w109:refnum<vi>)
        n74 = control-ref of="NO_EPV_122"() -> (w110:refnum<vi>)
        n75 = control-ref of="NC_EPV_61"() -> (w111:refnum<vi>)
        n76 = control-ref of="NC_EPV_1001"() -> (w112:refnum<vi>)
        n77 = control-ref of="F_EPV_1004"() -> (w113:refnum<vi>)
        n78 = control-ref of="F_EPV_1008"() -> (w114:refnum<vi>)
        n79 = control-ref of="N_EPV_1091"() -> (w115:refnum<vi>)
        n80 = control-ref of="NC_EPV_1217"() -> (w116:refnum<vi>)
        n81 = control-ref of="F_EPV_1007"() -> (w117:refnum<vi>)
        n82 = Build Array(w101, w102, w103, w104, w105, w106, w107, w108, w109, w110, w111, w112, w113, w114, w115, w116, w117) -> (w100:refnum<vi>[])
        n83 = call "SeCrTs-DO References FGV.vi"("State"=enum16{"Init", "Read", "Write"}."Write", "DO ref in"=w100) -> ()  [unwired: 8 in, 2 out]
      }
      frame "Initialize 3" {
        w130 = T7."Disabled and Grayed Out" ("Disabled")
        w137 = T12 [enum."Enabled", enum."Disabled and Grayed Out", enum."Disabled and Grayed Out", enum."Enabled", enum."Disabled and Grayed Out", enum."Disabled and Grayed Out", enum."Disabled and Grayed Out", enum."Enabled", enum."Enabled", enum."Enabled", enum."Enabled", enum."Disabled and Grayed Out", enum."Enabled", enum."Enabled", enum."Enabled", enum."Enabled", enum."Enabled", enum."Enabled", enum."Disabled and Grayed Out", enum."Enabled", enum."Enabled", enum."Enabled", enum."Enabled", enum."Enabled", enum."Enabled", enum."Disabled and Grayed Out", enum."Enabled", enum."Enabled", enum."Enabled", enum."Enabled"] items=["Enabled", "Disabled", "Disabled and Grayed Out"] ("Disabled")
        # "Enable /Disable"
        # "Enable/Disable"
        # "This case enable disable the control buttons"
        n84 = control-ref of="Connect RT"() -> (w141:refnum<vi>)
        n85 = control-ref of="START DAQ"() -> (w142:refnum<vi>)
        n86 = control-ref of="STOP DAQ"() -> (w143:refnum<vi>)
        n87 = control-ref of="DAQ SETTING"() -> (w144:refnum<vi>)
        n88 = control-ref of="START LOG"() -> (w145:refnum<vi>)
        n89 = control-ref of="STOP LOG"() -> (w146:refnum<vi>)
        n90 = control-ref of="HOLD UPDATE"() -> (w147:refnum<vi>)
        n91 = control-ref of="Connect Drive ATF"() -> (w148:refnum<vi>)
        n92 = control-ref of="Update drive ATF"() -> (w149:refnum<vi>)
        n93 = control-ref of="Gate driver ATF"() -> (w150:refnum<vi>)
        n94 = control-ref of="Motor On ATF"() -> (w151:refnum<vi>)
        n95 = control-ref of="Motor off ATF"() -> (w152:refnum<vi>)
        n96 = control-ref of="MCU reset ATF"() -> (w153:refnum<vi>)
        n97 = control-ref of="ADC reset ATF"() -> (w154:refnum<vi>)
        n98 = control-ref of="Connect ppsu"() -> (w155:refnum<vi>)
        n99 = control-ref of="update ppsu"() -> (w156:refnum<vi>)
        n100 = control-ref of="DC on"() -> (w157:refnum<vi>)
        n101 = control-ref of="Alarm ack"() -> (w158:refnum<vi>)
        n102 = control-ref of="DC off"() -> (w159:refnum<vi>)
        n103 = control-ref of="Ms initialize"() -> (w160:refnum<vi>)
        n104 = control-ref of="RT Stop"() -> (w161:refnum<vi>)
        n105 = control-ref of="ABORT"() -> (w162:refnum<vi>)
        n106 = control-ref of="Log type"() -> (w138:refnum<vi>)
        n107 = Build Array(w141, w142, w143, w144, w145, w146, w147, w148, w149, w150, w151, w152, w153, w154, w155, w156, w157, w158, w159, w160, w161, w162, w138) -> (w134:refnum<vi>[])
        n108 = control-ref of="PUMP IP"() -> (w131:refnum<vi>)
        n109 = control-ref of="STORAGE IP"() -> (w135:refnum<vi>)
        n110 = call "SeCrTs-enable disable malleable.vim"("error in"=w136, "Data"=w130, "Ref in"=w135) -> ("error out"=w133:errorcluster)  [unwired: 8 in]
        n111 = call "SeCrTs-enable disable malleable.vim"("error in"=w133, "Data"=w130, "Ref in"=w131) -> ("error out"=w132:errorcluster)  [unwired: 8 in]
        n112 = call "SeCrTs-enable disable malleable.vim"("Data"=w137, "Ref in"=w134) -> ()  [unwired: 9 in, 1 out]
      }
      frame "Initialize 4" {
        # "Cover screen  Visible?"
        # "User FGV"
        # "Log in"
        n113 = disable-structure shown="Disabled" {
          disable-tunnel: [w182 _] -> w174
          disable-tunnel: w172 -> [w181 _]
          frame Disabled {
            # "Call by ref"
            n114 = call "SeCrTs-File & Folder.vi"("error in (no error)"=w181) -> ("error out"=w177:errorcluster, "File Output"=w178:T11)  [unwired: 9 in]
            n115 = Unbundle By Name(w178) -> ("Sub vi's"=w180:path)
            n116 = Build Path(base path=w180, name or relative path=path "Login Main.vi") -> (appended path=w179:path)
            n117 = call "SeCrTs-Call by reference.vi"("error in"=w177, "vi path"=w179) -> ("error out"=w182:errorcluster)  [unwired: 9 in]
          }
          frame Enabled {
          }
        }
        n118 = Unbundle By Name(w171) -> ("Covers.Login screen cover"=w164:refnum<vi>, "Bol.DAQ SETTING"=w167:refnum<vi>)
        n119 = call "SeCrTs-User Details.vi"("Enum"=enum16{"Read", "Write"}."Read", "error in"=w174) -> ("error out"=w168:errorcluster, "User details R"=w175:string[])  [unwired: 8 in]
        n120 = Index Array(array=w175) -> (element #1=w169:string, element #2=→"User":string)  [unwired: 2 in]
        n121 = case shown="Default" w169 {
          tunnel: w168 -> [w183 w184 w185]
          tunnel: [w183 w184 w186] -> w166
          tunnel: w167 -> [_ _ w188]
          frame Default {
          }
          frame "Administrator" {
          }
          frame "Operator" {
            n122 = call "SeCrTs-enable disable malleable.vim"("error in"=w185, "Data"=T7."Disabled and Grayed Out" ("Disabled 2"), "Ref in"=w188) -> ("error out"=w186:errorcluster)  [unwired: 8 in]
          }
        }
        n123 = call "SeCrTs-enable disable malleable.vim"("error in"=w166, "Data"=FALSE, "Ref in"=w164) -> ("error out"=w165:errorcluster)  [unwired: 8 in]
      }
      frame "Ip Config" {
        # "This case will enable / Disable the IP address string"
        n124 = case shown="False" "Enable/Disable IP" {
          tunnel: w197 -> [w201 w203]
          tunnel: [w201 w203] -> w195
          tunnel: [T7."Disabled and Grayed Out" ("Disabled") T7."Enabled" ("Disabled")] -> w189
          frame False {
          }
          frame True {
          }
        }
        n125 = control-ref of="PUMP IP"() -> (w190:refnum<vi>)
        n126 = control-ref of="STORAGE IP"() -> (w194:refnum<vi>)
        n127 = call "SeCrTs-enable disable malleable.vim"("Data"=w189, "Ref in"=w190) -> ("error out"=w191:errorcluster)  [unwired: 9 in]
        n128 = call "SeCrTs-enable disable malleable.vim"("error in"=w195, "Data"=w189, "Ref in"=w194) -> ("error out"=w192:errorcluster)  [unwired: 8 in]
        n129 = Merge Errors(w191, w192) -> (w193:errorcluster)
      }
      frame "Start Daq" {
        # "This case will send the start daq command to the PXIe"
        n130 = Unbundle By Name(w207) -> ("Bol.START DAQ"=w215:refnum<vi>, "Bol.STOP DAQ"=w214:refnum<vi>, "Bol.START LOG"=w213:refnum<vi>, "Bol.STOP LOG"=w212:refnum<vi>, "Bol.HOLD UPDATE"=w211:refnum<vi>, "Bol.DAQ SETTING"=w210:refnum<vi>, "Bol.Exit RT"=w204:refnum<vi>)
        n131 = Build Array(w215, w214, w213, w212, w211, w210, w204) -> (w209:refnum<vi>[])
        n132 = case shown="Default" "Configuration File" {
          tunnel: w218 -> [w227 _]
          tunnel: w217 -> [w226 _]
          tunnel: w205 -> [w225 w229]
          tunnel: [w224 w229] -> w216
          tunnel: w209 -> [w221 _]
          frame Default {
            w220 = T12 [enum."Disabled and Grayed Out", enum."Enabled", enum."Enabled", enum."Disabled and Grayed Out", enum."Enabled", enum."Disabled and Grayed Out", enum."Disabled and Grayed Out"] items=["Enabled", "Disabled", "Disabled and Grayed Out"] ("Disabled")
            n133 = call "SeCrTs-NS Write.vi"("error in"=w225, "to"=enum16{"Storage", "Pumb", "Both"}."Both", "Data"=w227, "Message"=w226) -> ("error out"=w224:errorcluster)  [unwired: 7 in]
            n134 = call "SeCrTs-Stop Read FGV.vi"("Enum"=enum16{"Init", "Read", "Write"}."Write", "Stop"=FALSE) -> ()  [unwired: 9 in, 1 out]
            n135 = call "SeCrTs-enable disable malleable.vim"("Data"=w220, "Ref in"=w221) -> ()  [unwired: 9 in, 1 out]
          }
          frame "" {
            n136 = One Button Dialog(message="Please, Select the Configuration File !!") -> ()  [unwired: 1 in, 1 out]
          }
        }
      }
      frame "Close Connections" {
        # "This case will close the connection"
      }
      frame "Stop Daq" {
        # "This case will send the stop daq command to the PXIe"
        n137 = Unbundle By Name(w245) -> ("Bol.START DAQ"=w252:refnum<vi>, "Bol.STOP DAQ"=w251:refnum<vi>, "Bol.START LOG"=w250:refnum<vi>, "Bol.STOP LOG"=w249:refnum<vi>, "Bol.HOLD UPDATE"=w248:refnum<vi>, "Bol.DAQ SETTING"=w247:refnum<vi>, "Bol.Exit RT"=w244:refnum<vi>)
        n138 = call "SeCrTs-NS Write.vi"("error in"=w253, "to"=enum16{"Storage", "Pumb", "Both"}."Both", "Data"=w255, "Message"=w254) -> ("error out"=w241:errorcluster)  [unwired: 7 in]
        n139 = Build Array(w252, w251, w250, w249, w248, w247, w244) -> (w235:refnum<vi>[])
        n140 = call "SeCrTs-User Details.vi"("Enum"=enum16{"Read", "Write"}."Read", "error in"=w241) -> ("error out"=w240:errorcluster, "User details R"=w243:string[])  [unwired: 8 in]
        n141 = Index Array(array=w243) -> (element=w239:string)  [unwired: 1 in]
        n142 = case shown="\"Operator\"" w239 {
          tunnel: w240 -> [w257 w259]
          tunnel: [w257 w259] -> w238
          tunnel: [w256 w258] -> w234
          frame Default {
            w256 = T12 [enum."Enabled", enum."Disabled and Grayed Out", enum."Disabled and Grayed Out", enum."Disabled and Grayed Out", enum."Disabled and Grayed Out", enum."Enabled", enum."Enabled"] items=["Enabled", "Disabled", "Disabled and Grayed Out"] ("Disabled")
          }
          frame "Operator" {
            w258 = T12 [enum."Enabled", enum."Disabled and Grayed Out", enum."Disabled and Grayed Out", enum."Disabled and Grayed Out", enum."Disabled and Grayed Out", enum."Disabled and Grayed Out", enum."Enabled"] items=["Enabled", "Disabled", "Disabled and Grayed Out"] ("Disabled")
          }
        }
        n143 = call "SeCrTs-enable disable malleable.vim"("Data"=w234, "Ref in"=w235) -> ()  [unwired: 9 in, 1 out]
        n144 = call "SeCrTs-Stop Read FGV.vi"("Enum"=enum16{"Init", "Read", "Write"}."Write", "Stop"=TRUE) -> ()  [unwired: 9 in, 1 out]
      }
      frame "Phase code name" {
        # "This case sends the phase code name the PXIe"
        n145 = local read "Datalog phase code"() -> (w260:string)
        n146 = To Variant(anything=w260) -> (Variant=w268:variant)
        n147 = call "SeCrTs-NS Write.vi"("error in"=w270, "to"=enum16{"Storage", "Pumb", "Both"}."Both", "Data"=w268, "Message"=w269) -> ("error out"=w265:errorcluster)  [unwired: 7 in]
        n148 = call "SeCrTs-CS Phase code name.vi"("Enum"=enum16{"Read", "Write"}."Write", "error in"=w265, "Phase code W"=w260) -> ("error out"=w264:errorcluster)  [unwired: 7 in, 1 out]
        n149 = Bundle By Name(cluster=w261, "Log cmd.Log Name"=w260) -> (w262:T3)
      }
      frame "Log Option" {
        n150 = stacked-sequence {
          seq-local: [w282 _] -> [_ w296]
          seq-local: ["Log option" _] -> [_ w295]
          seq-local: [w280 _] -> [_ w294]
          tunnel: w277 -> [w280 _]
          tunnel: w276 -> [_ w293]
          tunnel: [_ w292] -> w275
          tunnel: [w279 _] -> w272
          tunnel: [w278 _] -> w271
          frame #0 {
            n151 = Unbundle By Name("Log option") -> ("Log type"=w279:bool, "Log Period(Min)"=w278:dbl)
            n152 = Format Into String(format string="%d", w278) -> (resulting string=w284:string)  [unwired: 2 in, 1 out]
            n153 = case shown="False" w279 {
              tunnel: w284 -> [w289 _]
              tunnel: [w288 "Continuous logging mode is enabled. Press okay to proceed." ("string")] -> w283
              frame False {
                n154 = call <vilib>:"Space Constant.vi"() -> ("String"=w286:string)
                n155 = Concatenate Strings("Periodical log mode with " ("string"), w289, w286, "minutes of log file size is enabled .Press okay to proceed." ("string")) -> (w288:string)
              }
              frame True {
              }
            }
            n156 = Two Button Dialog(message=w283) -> (T button?=w282:bool)  [unwired: 2 in]
          }
          frame #1 {
            n157 = case shown="True" w296 {
              tunnel: w295 -> [_ w307]
              tunnel: w294 -> [w297 w303]
              tunnel: [w297 w300] -> w292
              tunnel: w293 -> [_ w299]
              frame False {
              }
              frame True {
                n158 = in-place {
                  n159 = in-place-cluster #1(w307) -> ("Log type"=w312:bool, "Log Period(Min)"=w315:dbl)
                  n160 = Multiply(x=w315, y=60.0) -> (x*y=w313:dbl)
                  n161 = in-place-cluster #1("Log type"=w312, "Log Period(Min)"=w313) -> (w305:cluster{"Log type":bool, "Log Period(Min)":dbl})
                }
                n162 = To Variant(anything=w305) -> (Variant=w306:variant)
                n163 = call "SeCrTs-NS Write.vi"("error in"=w303, "to"=enum16{"Storage", "Pumb", "Both"}."Both", "Data"=w306, "Message"="Log Option") -> ("error out"=w302:errorcluster)  [unwired: 7 in]
                n164 = for {
                  shift-right: [w310] -> w300
                  shift-left: w302 -> [w311]
                  tunnel: string[] ["Phase code name", "Start Datalog"] -> [w309] mode=indexing
                  tunnel: w299 -> [w308]
                  n165 = call "Enqueue Message.vi"("error in (no error)"=w311, "Message"=w309, "Message Queue"=w308) -> ("error out"=w310:errorcluster)  [unwired: 7 in, 1 out]
                }
              }
            }
          }
        }
        n166 = Bundle By Name(cluster=w273, "Log cmd.C/NC"=w272, "Log cmd.Log min"=w271) -> (w274:T3)
      }
      frame "Start Datalog" {
        w316 = bool[] [TRUE, FALSE] ("Start Stop log")
        w328 = T12 [enum."Disabled and Grayed Out", enum."Disabled and Grayed Out", enum."Disabled and Grayed Out", enum."Enabled", enum."Enabled", enum."Disabled and Grayed Out"] items=["Enabled", "Disabled", "Disabled and Grayed Out"] ("Disabled")
        # "This case enable/Disable the log buttons and cover screens and sends the start log command to PXIe"
        n167 = Unbundle By Name(w325) -> ("Log cmd"=w324:refnum<notifier>)
        n168 = Unbundle By Name(w322) -> ("Bol.START DAQ"=w351:refnum<vi>, "Bol.STOP DAQ"=w350:refnum<vi>, "Bol.START LOG"=w349:refnum<vi>, "Bol.STOP LOG"=w348:refnum<vi>, "Bol.HOLD UPDATE"=w347:refnum<vi>, "Bol.Log type"=w333:refnum<vi>, "Covers"=w334:T13, "Log cmd"=w318:T14)
        n169 = call "SeCrTs-ALS Started FGV.vi"("Enum"=enum16{"Read", "Write"}."Read", "error in"=w340) -> ("error out"=w339:errorcluster, "Als started R"=w338:bool)  [unwired: 8 in]
        n170 = Concatenate Strings("Datalog phase code", "Trail Number") -> (w335:string)
        n171 = case shown="True" w338 {
          tunnel: [w353 w357] -> w317
          tunnel: w335 -> [w353 w355]
          tunnel: w339 -> [w352 w354]
          tunnel: [w352 w354] -> w321
          frame False {
            # "if sequence is nit"
          }
          frame True {
            # "If sequence started"
            n172 = Concatenate Strings("Auto " ("string"), "-" ("string"), w355) -> (w357:string)
          }
        }
        n173 = Build Array(w351, w350, w349, w348, w347, w333) -> (w329:refnum<vi>[])
        n174 = Unbundle(w334) -> ("cover"=w345:refnum<vi>, "Login screen cover"=w344:refnum<vi>, "cover Motor"=w343:refnum<vi>)
        n175 = Bundle By Name(cluster=w318, "Log Name"=w317, "Start/Stop Log"=w316) -> (w319:T14)
        n176 = Build Array(w345, w344, w343) -> (w327:refnum<vi>[])
        n177 = Send Notification(notification=w319, notifier=w324, error in (no error)=w321) -> (error out=w320:errorcluster)  [unwired: 1 out]
        n178 = call "SeCrTs-CS Start Stop Log.vi"("Enum"=enum16{"Read", "Write"}."Write", "error in"=w320, "Start Stop log"=w316) -> ("error out"=w332:errorcluster)  [unwired: 7 in, 1 out]
        n179 = Bundle By Name(cluster=w322, "Log cmd.Log Name"=w317, "Log cmd.Start/Stop Log"=w316) -> (w323:T3)
        n180 = call "SeCrTs-enable disable malleable.vim"("error in"=w332, "Data"=bool[] [FALSE, FALSE, FALSE, FALSE] ("Start Stop log"), "Ref in"=w327) -> ("error out"=w330:errorcluster)  [unwired: 8 in]
        n181 = call "SeCrTs-enable disable malleable.vim"("error in"=w330, "Data"=w328, "Ref in"=w329) -> ("error out"=w331:errorcluster)  [unwired: 8 in]
      }
      frame "Stop Datalog" {
        w359 = bool[] [FALSE, TRUE] ("Start Stop log")
        w373 = T12 [enum."Disabled and Grayed Out", enum."Enabled", enum."Enabled", enum."Disabled and Grayed Out", enum."Enabled", enum."Enabled"] items=["Enabled", "Disabled", "Disabled and Grayed Out"] ("Disabled")
        # "This case enable/Disable the log buttons and cover screens and sends the Stop log command to PXIe"
        n182 = Unbundle By Name(w365) -> ("Log cmd"=w364:refnum<notifier>)
        n183 = Unbundle By Name(w360) -> ("Bol.START DAQ"=w382:refnum<vi>, "Bol.STOP DAQ"=w386:refnum<vi>, "Bol.START LOG"=w385:refnum<vi>, "Bol.STOP LOG"=w384:refnum<vi>, "Bol.HOLD UPDATE"=w383:refnum<vi>, "Bol.Log type"=w375:refnum<vi>, "Covers"=w376:T13, "Log cmd"=w362:T14)
        n184 = Bundle By Name(cluster=w362, "Start/Stop Log"=w359) -> (w363:T14)
        n185 = Build Array(w382, w386, w385, w384, w383, w375) -> (w374:refnum<vi>[])
        n186 = Send Notification(notification=w363, notifier=w364, error in (no error)=w367) -> (error out=w366:errorcluster)  [unwired: 1 out]
        n187 = Unbundle(w376) -> ("cover"=w380:refnum<vi>, "Login screen cover"=w379:refnum<vi>, "cover Motor"=w378:refnum<vi>)
        n188 = call "SeCrTs-CS Start Stop Log.vi"("Enum"=enum16{"Read", "Write"}."Write", "error in"=w366, "Start Stop log"=w359) -> ("error out"=w372:errorcluster)  [unwired: 7 in, 1 out]
        n189 = Build Array(w380, w379, w378) -> (w370:refnum<vi>[])
        n190 = call "SeCrTs-enable disable malleable.vim"("error in"=w372, "Data"=bool[] [TRUE, FALSE, TRUE] ("Start Stop log"), "Ref in"=w370) -> ("error out"=w368:errorcluster)  [unwired: 8 in]
        n191 = Bundle By Name(cluster=w360, "Log cmd.Start/Stop Log"=w359) -> (w361:T3)
        n192 = call "SeCrTs-enable disable malleable.vim"("error in"=w368, "Data"=w373, "Ref in"=w374) -> ("error out"=w371:errorcluster)  [unwired: 8 in]
      }
      frame "Hold Update" {
        # "Hold Update"
        # "This case make hold the updation of Value updates on the monitoring screen"
        n193 = call "SeCrTs-Hold update .vi"("Enum"=enum16{"Read", "Write"}."Write", "error in (no error)"=w392, "In"="HOLD UPDATE") -> ("error out"=w391:errorcluster)  [unwired: 7 in, 1 out]
      }
      frame "Update Configuration" {
        # "This case update the configuration and send the configuration to the PXIe"
        n194 = call "SeCrTs-File & Folder.vi"("error in (no error)"=w404) -> ("error out"=w400:errorcluster, "File Output"=w403:T11)  [unwired: 9 in]
        n195 = local read "Configuration File"() -> (w401:string)
        n196 = Unbundle By Name(w403) -> ("Configuration path"=w402:path)
        n197 = Build Path(base path=w402, name or relative path=w401) -> (appended path=w397:path)
        n198 = Not A Number/Path/Refnum?(number/path/refnum=w397) -> (NaN/Path/Refnum?=w396:bool)
        n199 = case shown="False" w396 {
          tunnel: w397 -> [w417 _]
          tunnel: w400 -> [w416 w422]
          tunnel: [w412 w422] -> w399
          tunnel: [w405 _] -> w393
          frame False {
            # "If it is a path"
            n200 = Open/Create/Replace File(file path (use dialog)=w417, error in=w416, prompt="Select file to load", operation (0:open)=T9."open") -> (refnum out=w420:refnum<file>, error out=w415:errorcluster)  [unwired: 2 in, 1 out]
            n201 = Read from Binary File(5:T8 {"AO config"=[], "AI config"=[], "DI config"=[], "DO config"=[], "TC config"=[], "ACC config"=[], "SG config"=[], "Strain Gauge Settings"={"poisson ratio"=0.0, "nominal gage resistance"=120.0, "gage factor"=2.0}, "Bridge Settings"={"voltage excitation value"=3.0, "voltage excitation source"=10200, "initial bridge voltage"=0.0, "lead wire resistance"=1.7, "strain configuration"=10271}, "Sample Rate"={"AI Sample Rate"=[], "AO Sample Rate"=[], "DI Sample Rate"=[], "TC Sample Rate"=[], "DO Sample Rate"=[], "SG Sample Rate"=[], "ACC Sample Rate"=[]}} ("Data"), 8:w415, 11:w420) -> (0:w414:errorcluster, 2:w405:T8, 3:w421:refnum<file>)  [unwired: 3 in, 1 out]
            n202 = Close File(refnum=w421, error in=w414) -> (error out=w408:errorcluster)  [unwired: 1 out]
            n203 = call "SeCrTs-DO Search channel name.vi"("Data"=w405) -> ()  [unwired: 11 in]
            n204 = call "SeCrTs-DI Indexing.vi"("data"=w405) -> ()  [unwired: 11 in]
            n205 = call "SeCrTs-Configuration Data.vi"("Enum"=enum16{"Read", "Write"}."Write", "error in"=w408, "data"=w405) -> ("error out"=w407:errorcluster)  [unwired: 7 in, 1 out]
            n206 = To Variant(anything=w405) -> (Variant=w409:variant)
            n207 = call "SeCrTs-NS Write.vi"("error in"=w407, "to"=enum16{"Storage", "Pumb", "Both"}."Both", "Data"=w409, "Message"="Update Config") -> ("error out"=w412:errorcluster)  [unwired: 7 in]
          }
          frame True {
            # "Not a path"
          }
        }
        n208 = Bundle By Name(cluster=w394, "Log cmd.Config"=w393) -> (w395:T3)
      }
      frame "Write DO" {
        w432 = FALSE ("element")
        (unwired) FALSE  # Gate driver reset
        w427 = errorcluster {"status"=FALSE, "code"=0, "source"=""} ("error in")
        # "This case write the DO values and send the Data to PXIe"
        n209 = Build Array("NC_EPV_1211", "NO_EPV_1102", "NC_EPV_1214", "NC_EPV_1207", "AC_Switch") -> (w445:bool[])
        n210 = Build Array("F_EPV_1004", "F_EPV_1008", "N_EPV_1091", "NC_EPV_1217", "Gate driver ATF", w432, w432) -> (w428:bool[])
        n211 = To Variant(anything=w428) -> (Variant=w430:variant)
        n212 = To Variant(anything=w445) -> (Variant=w446:variant)
        n213 = call "SeCrTs-NS Write.vi"("error in"=w427, "to"=enum16{"Storage", "Pumb", "Both"}."Pumb", "Data"=w430, "Message"="Write DO") -> ("error out"=w425:errorcluster)  [unwired: 7 in]
        n214 = call "SeCrTs-NS Write.vi"("error in"=w427, "to"=enum16{"Storage", "Pumb", "Both"}."Storage", "Data"=w446, "Message"="Write DO") -> ("error out"=w426:errorcluster)  [unwired: 7 in]
        n215 = Merge Errors(w425, w426) -> (w424:errorcluster)
      }
      frame "Update Valve State" {
        # "HAVE to WORK on it"
        # "Valve Update"
        # "Configuration FGV"
        # "DO Reference FGV"
        # "This will update the valve status of the front panel based on the configuration"
        n216 = call "SeCrTs-DO References FGV.vi"("State"=enum16{"Init", "Read", "Write"}."Read") -> ("DO ref out"=w448:refnum<vi>[])  [unwired: 9 in, 1 out]
        n217 = call "SeCrTs-Configuration Data.vi"("Enum"=enum16{"Read", "Write"}."Read", "error in"=w454) -> ("error out"=w453:errorcluster, "data 2"=w451:T8)  [unwired: 8 in]
        n218 = call "SeCrTs-Do State extracter.vi"("error in"=w453, "input cluster"=w451, "EPV ref"=w448) -> ("error out"=w452:errorcluster)  [unwired: 8 in]
      }
      frame "Connect RT" {
        # "This case establish the connection to PXIe"
        n219 = Unbundle By Name(w472) -> ("Bol.Connect RT"=w470:refnum<vi>, "Bol.START DAQ"=w459:refnum<vi>)
        n220 = case shown="\"Both\", Default" "Select type" {
          tunnel: [w475 w480 w484] -> w467
          tunnel: [TRUE ("Storage rt con") TRUE ("Storage rt con") FALSE ("Storage rt con")] -> w465
          tunnel: "STORAGE IP" -> [w475 w480 w484]
          tunnel: "PUMP IP" -> [w474 w479 w483]
          tunnel: [w474 w479 w483] -> w462
          tunnel: [TRUE ("Pumb rt con") FALSE ("Pumb rt con") TRUE ("Pumb rt con")] -> w461
          frame "Both", Default {
          }
          frame "Storage" {
          }
          frame "Pump" {
          }
        }
        n221 = call "ATF-RT Con FGV.vi"("Storage rt con"=w465, "Enum"=enum16{"Read", "Write"}."Write", "Storage IP"=w467, "Pumb rt con"=w461, "Pump IP"=w462, "error in"=w460) -> ("Stoarge rt con R"=w458:bool, "error out"=w457:errorcluster)  [unwired: 5 in, 3 out]
        n222 = case shown="True" w458 {
          tunnel: T7."Disabled and Grayed Out" ("Disabled 2") -> [_ w489]
          tunnel: w470 -> [_ w488]
          tunnel: T7."Enabled" ("Disabled 2") -> [_ w487]
          tunnel: w459 -> [_ w486]
          frame False {
          }
          frame True {
            n223 = call "SeCrTs-enable disable malleable.vim"("Data"=w489, "Ref in"=w488) -> ()  [unwired: 9 in, 1 out]
            n224 = call "SeCrTs-enable disable malleable.vim"("Data"=w487, "Ref in"=w486) -> ()  [unwired: 9 in, 1 out]
          }
        }
      }
      frame "Set End Time" {
        # "Send T ZERO time to PXIe"
        # "This case send T zero data to the PXIe fo Sequence end time"
        n225 = To Variant(anything="T-0") -> (Variant=w497:variant)
        n226 = call "SeCrTs-NS Write.vi"("error in"=w496, "to"=enum16{"Storage", "Pumb", "Both"}."Both", "Data"=w497, "Message"="Set End Time") -> ("error out"=w493:errorcluster)  [unwired: 7 in]
      }
      frame "Get Sequence" {
        w502 = enum16{"SEQ", "CDT"}."CDT" ("Enum")
        # "Abort Sequence"
        # "This  case extract  the sequence data from the Sequenece file and send the data to the PXIe"
        n227 = call "SeCrTs-File & Folder.vi"("error in (no error)"=w524) -> ("error out"=w522:errorcluster, "File Output"=w523:T11)  [unwired: 9 in]
        n228 = Unbundle By Name(w523) -> ("Sequence"=w499:path)
        n229 = Build Path(base path=w499, name or relative path="SELECT SEQUENCER FILE") -> (appended path=w521:path)
        n230 = call "SeCrTs-Sequence Files Seperater.vi"("Array in"="SELECT ABORT SEQUENCE", "Sequence"=w499) -> ("Array"=w498:T15)  [unwired: 9 in]
        n231 = call "SeCrTs-Sequence separator.vi"("Sequence Folder Path"=w521, "error  in"=w522) -> ("AI"=w520:T16, "AO"=w519:T16, "DI"=w518:T16, "DO"=w517:T16, "error out"=w516:errorcluster)  [unwired: 9 in]
        n232 = call "SeCrTs-CDT DIVIDER.vi"("Enum"=w502, "Seq in"=w520) -> ("Array"=w515:T15)  [unwired: 9 in]
        n233 = call "SeCrTs-CDT DIVIDER.vi"("Enum"=w502, "Seq in"=w519) -> ("Array"=w514:T15)  [unwired: 9 in]
        n234 = call "SeCrTs-CDT DIVIDER.vi"("Enum"=w502, "Seq in"=w518) -> ("Array"=w513:T15)  [unwired: 9 in]
        n235 = call "SeCrTs-CDT DIVIDER.vi"("Enum"=w502, "Seq in"=w517) -> ("Array"=w512:T15)  [unwired: 9 in]
        n236 = To Variant(anything=w498) -> (Variant=w503:variant)
        n237 = To Variant(anything=w515) -> (Variant=w511:variant)
        n238 = To Variant(anything=w514) -> (Variant=w510:variant)
        n239 = To Variant(anything=w513) -> (Variant=w508:variant)
        n240 = To Variant(anything=w512) -> (Variant=w509:variant)
        n241 = Build Array(w503, w511, w510, w508, w509) -> (w507:variant[])
        n242 = for {
          tunnel: w507 -> [w529] mode=indexing
          tunnel: string[] ["Total Sequence", "Sequence Data AI", "Sequence Data AO", "Sequence Data DI", "Sequence Data DO"] -> [w528] mode=indexing
          shift-right: [w527] -> w504
          shift-left: w516 -> [w530]
          n243 = call "SeCrTs-NS Write.vi"("error in"=w530, "to"=enum16{"Storage", "Pumb", "Both"}."Both", "Data"=w529, "Message"=w528) -> ("error out"=w527:errorcluster)  [unwired: 7 in]
        }
      }
      frame "Start or Revert Sequence" {
        # "This acse send the start & revert  sequence command to the PXIe"
        n244 = Select(t="Start Sequence", s="Start or Revert Sequence", f="Revert Sequence") -> (s? t:f=w539:string)
        n245 = call "SeCrTs-NS Write.vi"("error in"=w538, "to"=enum16{"Storage", "Pumb", "Both"}."Both", "Message"=w539) -> ("error out"=w533:errorcluster)  [unwired: 8 in]
        n246 = call "SeCrTs-DO References FGV.vi"("State"=enum16{"Init", "Read", "Write"}."Read", "error in"=w533) -> ("error out"=w532:errorcluster, "DO ref out"=w534:refnum<vi>[])  [unwired: 8 in]
        n247 = case shown="False" "Start or Revert Sequence" {
          tunnel: w532 -> [w545 w551]
          tunnel: [w544 w550] -> w535
          tunnel: w534 -> [w547 w549]
          frame False {
            n248 = call "SeCrTs-enable disable malleable.vim"("error in"=w545, "Data"=T7."Enabled" ("Disabled 2"), "Ref in"=w547) -> ("error out"=w544:errorcluster)  [unwired: 8 in]
          }
          frame True {
            n249 = call "SeCrTs-enable disable malleable.vim"("error in"=w551, "Data"=T7."Disabled" ("Disabled 2"), "Ref in"=w549) -> ("error out"=w550:errorcluster)  [unwired: 8 in]
          }
        }
      }
      frame "Hold CDT" {
        # "This case sends the Hold & Release Command to the PXIe to hold or Release  the timer"
        n250 = Select(t="Hold CDT", s="HOLD CDT", f="Release CDT") -> (s? t:f=w556:string)
        n251 = To Variant(anything="HOLD CDT") -> (Variant=w555:variant)
        n252 = call "SeCrTs-NS Write.vi"("error in"=w560, "to"=enum16{"Storage", "Pumb", "Both"}."Both", "Data"=w555, "Message"=w556) -> ("error out"=w559:errorcluster)  [unwired: 7 in]
      }
      frame "Connect Drive ATF" {
        # "Establish connection to the ATF Drive"
        n253 = To Variant(anything=TRUE) -> (Variant=w565:variant)
        n254 = call "SeCrTs-NS Write.vi"("error in"=w566, "to"=enum16{"Storage", "Pumb", "Both"}."Pumb", "Data"=w565, "Message"=w564) -> ("error out"=w563:errorcluster)  [unwired: 7 in]
      }
      frame "Update Drive ATF Values" {
        # "Updates all the values to the ATF Drive"
        n255 = flat-sequence {
          tunnel: w572 -> [w579]
          tunnel: [w578] -> w571
          tunnel: w571 -> [w587]
          tunnel: [w587] -> w570
          frame #0 {
            n256 = Build Array("SET FREQ", "RAMP UP", "RAMP DOWN", "SPEED", 0.0 ("element")) -> (w581:dbl[])
            n257 = property on="State ATF" class="Knob (strict)"("Scale.Maximum"="SPEED") -> ()  [unwired: 2 in, 2 out]
            n258 = Array To Cluster(array=w581) -> (cluster=w580:T17)
            n259 = To Variant(anything=w580) -> (Variant=w577:variant)
            n260 = call "SeCrTs-NS Write.vi"("error in"=w579, "to"=enum16{"Storage", "Pumb", "Both"}."Pumb", "Data"=w577, "Message"="Update Drive ATF") -> ("error out"=w578:errorcluster)  [unwired: 7 in]
          }
          frame #1 {
            n261 = One Button Dialog(message="The ATF Drive set parameters are updated .") -> ()  [unwired: 1 in, 1 out]
          }
        }
      }
      frame "Gate Driver Power ATF" {
        # "Trigger Gate driver power"
        n262 = call "SeCrTs-NS Write.vi"("error in"=w593, "to"=enum16{"Storage", "Pumb", "Both"}."Pumb", "Data"=w591, "Message"=w592) -> ("error out"=w590:errorcluster)  [unwired: 7 in]
      }
      frame "ADC Reset ATF" {
        # "Reset ADC of Drive ATF"
      }
      frame "MCU Reset ATF" {
        # "This case reset the MCU of ATF Drive"
      }
      frame "Motor On ATF" {
        w606 = T12 [enum."Disabled and Grayed Out", enum."Disabled and Grayed Out", enum."Disabled and Grayed Out", enum."Disabled and Grayed Out", enum."Disabled and Grayed Out", enum."Enabled"] items=["Enabled", "Disabled", "Disabled and Grayed Out"] ("Disabled")
        # "sends Motor ON command to the ATF Motor"
        n263 = Unbundle By Name(w608) -> ("Bol.Update drive ATF"=w615:refnum<vi>, "Bol.Gate driver ATF"=w614:refnum<vi>, "Bol.ADC reset ATF"=w613:refnum<vi>, "Bol.MCU reset ATF"=w612:refnum<vi>, "Bol.Motor On ATF"=w611:refnum<vi>, "Bol.Motor off ATF"=w610:refnum<vi>)
        n264 = Build Array(w615, w614, w613, w612, w611, w610) -> (w607:refnum<vi>[])
        n265 = call "SeCrTs-enable disable malleable.vim"("Data"=w606, "Ref in"=w607) -> ()  [unwired: 9 in, 1 out]
        n266 = call "SeCrTs-NS Write.vi"("error in"=w603, "to"=enum16{"Storage", "Pumb", "Both"}."Pumb", "Message"="Motor On ATF") -> ("error out"=w602:errorcluster)  [unwired: 8 in]
      }
      frame "Motor Off ATF" {
        w620 = T12 [enum."Enabled", enum."Enabled", enum."Enabled", enum."Enabled", enum."Enabled", enum."Disabled and Grayed Out"] items=["Enabled", "Disabled", "Disabled and Grayed Out"] ("Disabled")
        # "sends Motor OFF command to the ATF Motor"
        n267 = Unbundle By Name(w623) -> ("Bol.Update drive ATF"=w629:refnum<vi>, "Bol.Gate driver ATF"=w628:refnum<vi>, "Bol.ADC reset ATF"=w627:refnum<vi>, "Bol.MCU reset ATF"=w626:refnum<vi>, "Bol.Motor On ATF"=w625:refnum<vi>, "Bol.Motor off ATF"=w624:refnum<vi>)
        n268 = Build Array(w629, w628, w627, w626, w625, w624) -> (w621:refnum<vi>[])
        n269 = call "SeCrTs-enable disable malleable.vim"("Data"=w620, "Ref in"=w621) -> ()  [unwired: 9 in, 1 out]
        n270 = call "SeCrTs-NS Write.vi"("error in"=w617, "to"=enum16{"Storage", "Pumb", "Both"}."Pumb", "Message"="Motor Off ATF") -> ("error out"=w616:errorcluster)  [unwired: 8 in]
      }
      frame "Connect PPSU" {
        # "This case establish the Conection to PPSU"
        n271 = call "SeCrTs-Connect PPSU.vi"("error In"=w632) -> ("error out"=w631:errorcluster)  [unwired: 10 in]
      }
      frame "DC ON PPSU" {
        w634 = T12 [enum."Disabled and Grayed Out", enum."Disabled and Grayed Out", enum."Disabled and Grayed Out", enum."Disabled and Grayed Out", enum."Enabled"] items=["Enabled", "Disabled", "Disabled and Grayed Out"] ("Disabled")
        # "PPSU DC Power ON"
        n272 = Unbundle By Name(w637) -> ("Bol.update ppsu"=w644:refnum<vi>, "Bol.Alarm ack"=w643:refnum<vi>, "Bol.Ms initialize"=w642:refnum<vi>, "Bol.DC on"=w641:refnum<vi>, "Bol.DC off"=w640:refnum<vi>)
        n273 = Build Array(w644, w643, w642, w641, w640) -> (w635:refnum<vi>[])
        n274 = call "SeCrTs-DC ON PPSU.vi"("Error in"=w639) -> ("Fehler (Ausgang)"=w638:errorcluster)  [unwired: 10 in]
        n275 = call "SeCrTs-enable disable malleable.vim"("Data"=w634, "Ref in"=w635) -> ()  [unwired: 9 in, 1 out]
      }
      frame "DC OFF PPSU" {
        w645 = T12 [enum."Enabled", enum."Enabled", enum."Enabled", enum."Enabled", enum."Disabled and Grayed Out"] items=["Enabled", "Disabled", "Disabled and Grayed Out"] ("Disabled")
        # "PPSU DC Power OFF"
        n276 = Unbundle By Name(w650) -> ("Bol.update ppsu"=w655:refnum<vi>, "Bol.Alarm ack"=w654:refnum<vi>, "Bol.Ms initialize"=w653:refnum<vi>, "Bol.DC on"=w652:refnum<vi>, "Bol.DC off"=w651:refnum<vi>)
        n277 = Build Array(w655, w654, w653, w652, w651) -> (w646:refnum<vi>[])
        n278 = call "SeCrTs-DC OFF PPSU.vi"("Error in"=w648) -> ("Fehler (Ausgang)"=w647:errorcluster)  [unwired: 10 in]
        n279 = call "SeCrTs-enable disable malleable.vim"("Data"=w645, "Ref in"=w646) -> ()  [unwired: 9 in, 1 out]
      }
      frame "Update PPSU Values" {
        # "This case updates the all PPSU values"
        n280 = flat-sequence {
          tunnel: w660 -> [w662]
          tunnel: [w661] -> w659
          tunnel: [w671] -> w658
          tunnel: w659 -> [w671]
          frame #0 {
            n281 = Bundle By Name(cluster=T10 {"OPP(W)"=0.0, "OVP(V)"=0.0, "OCP(A)"=0.0, "SET VOLTAGE"=0.0, "SET CURRENT"=0.0, "SET POWER"=0.0} ("Cluster"), "OPP(W)"="OPP(W)", "OVP(V)"="OVP(V)", "OCP(A)"="OCP(A)", "SET VOLTAGE"="SET VOLTAGE", "SET CURRENT"="SET CURRENT", "SET POWER"="SET POWER") -> (w663:T10)
            n282 = call "SeCrTs-Update PPSU Settings.vi"("Error in"=w662, "Cluster"=w663) -> ("Fehler (Ausgang)"=w661:errorcluster)  [unwired: 9 in]
          }
          frame #1 {
            n283 = One Button Dialog(message="The PPSU set parameters are updated.") -> ()  [unwired: 1 in, 1 out]
          }
        }
      }
      frame "Alarm Ack PPSU" {
        # "This case will acknowlede the PPSU alarm"
        n284 = call "SeCrTs-Alarm Ack PPSU.vi"("Error in"=w674) -> ("Fehler (Ausgang)"=w673:errorcluster)  [unwired: 10 in]
      }
      frame "MS Initialize PPSU" {
        # "This initialize the PPSU master Slave"
        n285 = call "SeCrTs-Master Slave Initialize PPSU.vi"("Error in"=w678) -> ("Fehler (Ausgang)"=w677:errorcluster)  [unwired: 10 in]
      }
      frame "RT Exit" {
        # "This Case EXIT  the RT"
        n286 = To Variant(anything=TRUE) -> (Variant=w685:variant)
        n287 = call "SeCrTs-NS Write.vi"("error in"=w686, "to"=enum16{"Storage", "Pumb", "Both"}."Both", "Data"=w685, "Message"=w687) -> ("error out"=w688:errorcluster)  [unwired: 7 in]
      }
      frame "RT Stop" {
        # "This Case occationally stops the RT"
        n288 = call "ATF-RT Con FGV.vi"("Enum"=enum16{"Read", "Write"}."Write") -> ()  [unwired: 10 in, 5 out]
        n289 = disable-structure shown="Disabled" {
          disable-tunnel: [w698 _] -> w693
          disable-tunnel: w690 -> [w697 _]
          frame Disabled {
            n290 = To Variant(anything=TRUE) -> (Variant=w696:variant)
            n291 = call "SeCrTs-NS Write.vi"("error in"=w697, "Data"=w696, "Message"="RT Stop") -> ("error out"=w698:errorcluster)  [unwired: 8 in]
          }
          frame Enabled {
          }
        }
      }
      frame "Exit" {
        w711 = enum16{"Init", "Read", "Write"}."Write" ("Enum")
        # "Exit"
        # "Stop Read"
        # "Loop EXIT and closes the reference"
        n292 = Unbundle By Name(w719) -> ("Storage Data"=w718:refnum<notifier>, "Pumb Data"=w699:refnum<notifier>)
        n293 = call "SeCrTs-NS Write.vi"("error in"=w717, "to"=enum16{"Storage", "Pumb", "Both"}."Both", "Message"=w715) -> ("error out"=w716:errorcluster)  [unwired: 8 in]
        n294 = call "Fire User Event - Stop.vi"("error in (no error)"=w716, "User Event - Stop"=w714) -> ("error out"=w701:errorcluster)  [unwired: 9 in]
        n295 = Release Notifier(notifier=w699, error in (no error)=w701) -> (error out=w700:errorcluster)  [unwired: 1 in, 2 out]
        n296 = Release Notifier(notifier=w718, error in (no error)=w700) -> (error out=w709:errorcluster)  [unwired: 1 in, 2 out]
        n297 = Release Queue(queue=w708, error in (no error)=w709) -> (error out=w707:errorcluster)  [unwired: 1 in, 2 out]
        n298 = Release Queue(queue=w706, error in (no error)=w707) -> (error out=w705:errorcluster)  [unwired: 1 in, 2 out]
        n299 = call "SeCrTs-Exit FGV.vi"("Enum"=w711, "Exit"=TRUE) -> ()  [unwired: 8 in, 2 out]
        n300 = call "SeCrTs-Stop Read FGV.vi"("Enum"=w711, "Stop"=TRUE) -> ()  [unwired: 9 in, 1 out]
        n301 = Release Queue(queue=w704, error in (no error)=w705) -> (error out=w703:errorcluster)  [unwired: 1 in, 2 out]
      }
      frame "Exit Drive ATF" {
        # "Exit ATF Drive"
        n302 = To Variant(anything=TRUE) -> (Variant=w724:variant)
        n303 = call "SeCrTs-NS Write.vi"("error in"=w728, "to"=enum16{"Storage", "Pumb", "Both"}."Pumb", "Data"=w724, "Message"=w726) -> ("error out"=w727:errorcluster)  [unwired: 7 in]
      }
      frame "Daq Setting" {
        # "Calls the daq setting VI Dynamically and updates the values to the sequence file"
        n304 = call "SeCrTs-File & Folder.vi"("error in (no error)"=w745) -> ("error out"=w744:errorcluster, "File Output"=w743:T11)  [unwired: 9 in]
        n305 = Unbundle By Name(w743) -> ("Configuration path"=w737:path, "Sub vi's"=w742:path)
        n306 = Build Path(base path=w742, name or relative path=path "SeCrTs-Hardware Config.vi") -> (appended path=w740:path)
        n307 = call "SeCrTs-Call by reference.vi"("error in"=w744, "vi path"=w740) -> ("error out"=w738:errorcluster)  [unwired: 9 in]
        n308 = List Folder(path=w737, error in=w738) -> (filenames=w729:string[], error out=w734:errorcluster)  [unwired: 2 in, 2 out]
        n309 = control-ref of="Configuration File"() -> (w739:refnum<vi>)
        n310 = call "SeCrTs-Configuration File Name.vi"("Enum"=enum16{"Read", "Write"}."Read", "error in"=w734) -> ("error out"=w733:errorcluster, "Phase codeR"=w730:string)  [unwired: 8 in]
        n311 = property on="Property Node" class="CmbBox"(reference=w739, error in=w733, "Value"=w730, "Strings[]"=w729) -> (error out=w736:errorcluster)  [unwired: 1 out]
      }
      frame "Abort" {
      }
      frame "Add User" {
        n312 = call "SeCrTs-File & Folder.vi"("error in (no error)"=w750) -> ("error out"=w755:errorcluster, "File Output"=w754:T11)  [unwired: 9 in]
        n313 = Unbundle By Name(w754) -> ("Sub vi's"=w753:path)
        n314 = Build Path(base path=w753, name or relative path=path "Add User.vi") -> (appended path=w752:path)
        n315 = call "SeCrTs-Call by reference.vi"("error in"=w755, "vi path"=w752) -> ("error out"=w749:errorcluster)  [unwired: 9 in]
      }
    }
    n316 = call "SeCrTs-Error handler P3.vi"("error in"=w41, "Message Queue"=w39) -> ("error out"=w40:errorcluster)  [unwired: 8 in, 1 out]
  }
  n317 = while {
    tunnel: w29 -> [w831]
    tunnel: w15 -> [w785]
    tunnel: w5 -> [w783]
    stop <- w830 stop-if-true
    w781 = 100 ("timeout in ms (-1)")
    # "String Display"
    # "Sequence Status"
    # "Do Display"
    # "RT Error Display"
    # "PPSU Health"
    # "Health Status"
    # "Log Health"
    # "CDT Display"
    # "CS Error Display"
    # "Drive LOX"
    # "ATF Drive"
    # "PPSU"
    # "Monitoring Loop"
    n318 = call "SeCrTs-Error FGV  RT.vi"("Enum"=enum16{"Read", "Write", "Clear"}."Read") -> ("CS err"=w792:T18)  [unwired: 10 in]
    n319 = call "SeCrTs-Error FGV.vi"("Enum"=enum16{"Read", "Write", "Clear"}."Read") -> ("CS err"=w795:T18)  [unwired: 10 in]
    n320 = Wait on Notification(notifier=w831, timeout in ms (-1)=w781) -> (notification=w828:T19, error out=w797:errorcluster)  [unwired: 2 in, 2 out]
    n321 = Wait on Notification(notifier=w783, timeout in ms (-1)=w781) -> (notification=w780:T19, error out=w782:errorcluster)  [unwired: 2 in, 2 out]
    n322 = Unbundle By Name(w792) -> ("Error Source"=→"PXIe Error Display":string)
    n323 = Unbundle By Name(w795) -> ("Error Source"=→"Control Screen Error Display":string)
    n324 = call "SSeCrT-seq Execution Monitor  HOST.vi"("Enum"=enum16{"Read", "Write "}."Read") -> ("Seq Monitor Out"=w788:string[])  [unwired: 9 in, 1 out]
    n325 = call "SeCrTs-PPSU Health.vi"("Enum"=enum16{"Read", "Write"}."Read") -> ("ppsu health R"=→"PPSU Health":bool)  [unwired: 9 in, 1 out]
    n326 = call "SeCrTs-PPSU Feedback.vi"("PPSU Queue"=w785, "Enable PPSU"="Connect ppsu") -> ("Power"=→"Terminal Power":i32, "Current"=→"Terminal Current":i32, "Voltage"=→"Terminal Voltage":i32, "Fault Status"=w817:bool[], "No .of slaves"=→"No .of Slaves":u8)  [unwired: 4 in, 1 out]
    n327 = Compound Arithmetic op=OR(w797, "Exit", w782) -> (w830:bool)
    n328 = Index Array(array=w817) -> (element #2=→"power failure status":bool, element #3=→"MS failure":bool, element #4=→"over voltage detection":bool, element #5=→"Over current detection":bool, element #6=→"Over power detection":bool)  [unwired: 6 in, 1 out]
    n329 = call "SeCrTs-Seq Display.vi"("Seq Monitor"=w788) -> ("out"=→"SEQUENCE STATE":string)  [unwired: 9 in, 1 out]
    n330 = Unbundle By Name(w828) -> ("DI_Data"=w778:digitalwaveform[], "DO"=w790:waveform(dbl)[], "Loop Status"=w762:bool[])
    n331 = Unbundle By Name(w780) -> ("DI_Data"=w779:digitalwaveform[], "Loop Status"=w766:bool[])
    n332 = call "SeCrTs-DI Search Channel.vi"("DI Data"=w779) -> ("Array 2"=w772:bool[])  [unwired: 10 in]
    n333 = call "SeCrTs-DO Data display.vi"("DO"=w790) -> ()  [unwired: 11 in]
    n334 = Index Array(array=w772) -> (element #1=→"F_EPV_1004_HSS":bool, element #2=→"F_EPV_1008_HSS":bool, element #3=→"N_EPV_1091_HSS":bool, element #4=→"NC_EPV_1217_HSS":bool)  [unwired: 4 in]
    n335 = Index Array(array=w766) -> (element #1=→"AI C Health":bool, element #2=→"AI V Health":bool, element #3=→"AO Health":bool, element #4=→"DI Health":bool, element #5=→"DO Health":bool, element #6=→"TC Health":bool, element #7=→"ACC Health":bool, element #9=→"Drive ATF Health":bool)  [unwired: 9 in, 1 out]
    n336 = Get Date/Time In Seconds() -> (seconds since 1Jan1904=→"Time":timestamp)
    n337 = call "ATF-DI Display Filtyer.vi"("DI Data"=w778) -> ("DI out"=w777:bool[])  [unwired: 10 in]
    n338 = Index Array(array=w777) -> (element #1=→"NO_EPV_1102_HSS":bool, element #2=→"NC_EPV_1211_HSS":bool, element #3=→"NC_EPV_1214_HSS":bool, element #4=→"NC_EPV_1207_HSS":bool)  [unwired: 4 in]
    n339 = call "SeCrTs-CDT.vi"("Write/Read"=enum16{"Write", "Read"}."Read") -> ("CDT Out"=w800:dbl)  [unwired: 9 in, 1 out]
    "COUNT DOWN TIMER" <- w800
    n340 = Index Array(array=w762, index #2=3 ("index"), index #3=0 ("index"), index #4=7 ("index")) -> (element #1=→"AI C Health  S":bool, element #2=→"DI Health S":bool, element #3=→"DO Health S":bool, element #4=→"Target":bool)  [unwired: 1 in]
    n341 = Greater Than 0?(x=w800) -> (x > 0?=w799:bool)
    n342 = Select(t="%<+%H:%M:%S%3u>t", s=w799, f="%<%H:%M:%S%3u>t") -> (s? t:f=w805:string)
    n343 = property on="COUNT DOWN TIMER" class="DigNum (strict)"("FormatString"=w805) -> ()  [unwired: 2 in, 2 out]
    n344 = call "SeCrTs-RT Connected .vi"("Enum"=enum16{"Read", "Write"}."Read") -> ("Pumb rt con R"=→"Target 2":bool)  [unwired: 8 in, 2 out]
    n345 = call "SeCrTs-CS Log Health.vi"("Enum"=enum16{"Read", "Write"}."Read") -> ("Log health R"=→"Log?":bool)  [unwired: 9 in, 1 out]
    "Rotational sate" <- "-------" ("User 2")
  }
  n346 = call "ATF-Pump NS Main.vi"("Queues"=w3, "Pump DP"=w2) -> ()  [unwired: 10 in]
  n347 = call "ATF-Storage NS Main.vi"("Queues"=w3, "Data"=w14) -> ()  [unwired: 9 in, 1 out]
  n348 = call "SeCrTs-Event logger.vi"(11:w3) -> ()  [unwired: 11 in]
  n349 = call "SeCrTs-Error logger RT Pumb.vi"(11:w3) -> ()  [unwired: 11 in]
  n350 = call "SeCrTs-Error logger RT Storage.vi"(11:w3) -> ()  [unwired: 11 in]
  n351 = call "SeCrTs-Error logger.vi"(11:w3) -> ()  [unwired: 11 in]
  n352 = call "SeCrTs-CS Queue Data log module.vi"(11:w3) -> ()  [unwired: 10 in, 1 out]
  n353 = call "ATF-Log command to DR.vi"("Cluster"=w4) -> ()  [unwired: 10 in, 1 out]
  n354 = call "ATF-Log command to DD.vi"("Cluster"=w4) -> ()  [unwired: 10 in, 1 out]
  n355 = while {
    tunnel: w36 -> [w844]
    tunnel: [w843] -> w35
    tunnel: w18 -> [w842]
    shift-right: [w833] -> w31
    shift-left: _ -> [w841]
    tunnel: w13 -> [w837]
    tunnel: w17 -> [w832]
    stop <- w838 stop-if-true
    # "Error handler"
    # "Event Driven Loop"
    n356 = event shown="[33] \"RT Stop\": Value Change" {
      selector: w844 -> [_ _ _ _ _ _ _ _ _ _ _ _ _ _ _ _ _ _ _ _ _ _ _ _ _ _ _ _ _ _ _ _ _ _ _]
      dyn-events: [_ _ _ _ _ _ _ _ _ _ _ _ _ _ _ _ _ _ _ _ _ _ _ _ _ _ _ _ _ _ _ _ _ _ _] -> w843
      timeout: _ -> [_ _ _ _ _ _ _ _ _ _ _ _ _ _ _ _ _ _ _ _ _ _ _ _ _ _ _ _ _ _ _ _ _ _ _]
      tunnel: [FALSE FALSE FALSE FALSE FALSE _ FALSE FALSE FALSE FALSE FALSE FALSE TRUE FALSE FALSE FALSE FALSE FALSE FALSE FALSE FALSE FALSE FALSE FALSE FALSE FALSE FALSE FALSE FALSE FALSE FALSE FALSE FALSE FALSE FALSE] -> w839
      tunnel: w842 -> [w858 w864 w870 w878 w889 w902 w910 w922 w930 w936 w950 w956 w960 w968 w973 w982 w991 w998 w1005 w1009 w1016 w1023 w1030 w1038 w1045 w1051 w1059 w1064 w1073 w1080 w1087 w1094 w1101 w1108 w1117]
      tunnel: w841 -> [w857 w865 w872 w879 w891 w901 w911 w924 w931 w938 w949 w958 w959 w965 w975 w981 w989 w997 w1004 w1012 w1018 w1026 w1032 w1040 w1047 w1053 w1061 w1067 w1075 w1082 w1089 w1096 w1103 w1110 w1116]
      tunnel: [w857 w861 w871 w877 w881 w901 w917 w923 w929 w942 w948 w957 w959 w966 w974 w980 w988 w996 w1003 w1011 w1017 w1025 w1031 w1039 w1046 w1052 w1060 w1066 w1074 w1081 w1088 w1095 w1102 w1109 w1115] -> w836
      tunnel: [w858 w862 w868 w876 w895 w902 w915 w921 w928 w940 w947 w955 w960 w967 w972 w979 w987 w995 w1002 w1010 w1015 w1024 w1029 w1037 w1044 w1050 w1058 w1065 w1072 w1079 w1086 w1093 w1100 w1107 w1114] -> w840
      tunnel: [_ w859 w866 w873 w892 w900 w903 w919 w926 w932 w943 w952 _ w962 w969 w976 w983 w992 w999 w1006 w1013 w1020 w1027 w1034 w1041 w1048 w1055 w1062 w1069 w1076 w1083 w1090 w1097 w1104 w1111] -> w835
      event Timeout {
        n357 = event-data() -> ()  [unwired: 1 in, 3 out]
      }
      event "SET": Value Change {
        n358 = event-data() -> ("CtlRef"=w859:refnum<vi>)  [unwired: 1 in]
        n359 = call "Enqueue Message.vi"("error in (no error)"=w865, "Message"="Set End Time", "Message Queue"=w864) -> ("error out"=w861:errorcluster, "dup Message Queue"=w862:refnum<queue>)  [unwired: 7 in]
      }
      event "NO_EPV_122", "NC_EPV_61", "NC_EPV_1001", "NC_EPV_1211", "NO_EPV_1102", "NC_EPV_1214", "NC_EPV_1207", "AC_Switch", "NC_EPV_481", "NO_EPV_478R", "NO_EPV_477", "NC_EPV_56", "F_EPV_1004", "N_EPV_1091", "F_EPV_1007", "F_EPV_1008", "NC_EPV_1217": Value Change {
        n360 = event-data() -> ("CtlRef"=w866:refnum<vi>)  [unwired: 1 in]
        n361 = call "Enqueue Message.vi"("error in (no error)"=w872, "Message"="Write DO", "Message Queue"=w870) -> ("error out"=w871:errorcluster, "dup Message Queue"=w868:refnum<queue>)  [unwired: 7 in]
      }
      event "Get Sequence": Value Change {
        n362 = event-data() -> ("CtlRef"=w873:refnum<vi>)  [unwired: 1 in]
        n363 = call "Enqueue Message.vi"("error in (no error)"=w879, "Message"="Get Sequence", "Message Queue"=w878) -> ("error out"=w877:errorcluster, "dup Message Queue"=w876:refnum<queue>)  [unwired: 7 in]
      }
      event "Start or Revert Sequence": Value Change {
        n364 = event-data() -> ("NewVal"=w880:bool, "CtlRef"=w892:refnum<vi>)  [unwired: 1 in]
        n365 = call "Enqueue Message.vi"("error in (no error)"=w891, "Message"="Stop Datalog", "Message Queue"=w889) -> ("error out"=w885:errorcluster, "dup Message Queue"=w884:refnum<queue>)  [unwired: 7 in]
        n366 = call "Enqueue Message.vi"("error in (no error)"=w885, "Message"="Start Datalog", "Message Queue"=w884) -> ("error out"=w890:errorcluster, "dup Message Queue"=w888:refnum<queue>)  [unwired: 7 in]
        n367 = call "Enqueue Message.vi"("error in (no error)"=w890, "Message"="Start or Revert Sequence", "Message Queue"=w888) -> ("error out"=w882:errorcluster, "dup Message Queue"=w895:refnum<queue>)  [unwired: 7 in]
        n368 = call "SeCrTs-ALS Started FGV.vi"("Enum"=enum16{"Read", "Write"}."Write", "error in"=w882, "Als started?"=w880) -> ("error out"=w881:errorcluster)  [unwired: 7 in, 1 out]
      }
      event "Log option": Value Change {
        n369 = event-data() -> ("CtlRef"=w900:refnum<vi>, "NewVal.Log type"=w896:bool)  [unwired: 1 in]
        n370 = Select(t=T7."Disabled and Grayed Out" ("Disabled"), s=w896, f=T7."Enabled") -> (s? t:f=w899:T7)
        n371 = property on="Log Period(Min)" class="DigNum (strict)"("DisabledEnum"=w899) -> ()  [unwired: 2 in, 2 out]
      }
      event "START DAQ": Value Change {
        n372 = event-data() -> ("CtlRef"=w903:refnum<vi>)  [unwired: 1 in]
        n373 = call "Enqueue Message.vi"("error in (no error)"=w911, "Message"="Update Configuration", "Message Queue"=w910) -> ("error out"=w908:errorcluster, "dup Message Queue"=w907:refnum<queue>)  [unwired: 7 in]
        n374 = call "Enqueue Message.vi"("error in (no error)"=w908, "Message"="Update Valve State", "Message Queue"=w907) -> ("error out"=w905:errorcluster, "dup Message Queue"=w906:refnum<queue>)  [unwired: 7 in]
        n375 = To Variant(anything=bool[] [TRUE, FALSE]) -> (Variant=w913:variant)
        n376 = call "Enqueue Message.vi"("error in (no error)"=w905, "Message Data"=w913, "Message"="Start Daq", "Message Queue"=w906) -> ("error out"=w917:errorcluster, "dup Message Queue"=w915:refnum<queue>)  [unwired: 6 in]
      }
      event "HOLD CDT": Value Change {
        n377 = event-data() -> ("CtlRef"=w919:refnum<vi>)  [unwired: 1 in]
        n378 = call "Enqueue Message.vi"("error in (no error)"=w924, "Message"="Hold CDT", "Message Queue"=w922) -> ("error out"=w923:errorcluster, "dup Message Queue"=w921:refnum<queue>)  [unwired: 7 in]
      }
      event "START LOG": Value Change {
        n379 = event-data() -> ("CtlRef"=w926:refnum<vi>)  [unwired: 1 in]
        n380 = call "Enqueue Message.vi"("error in (no error)"=w931, "Message"="Log Option", "Message Queue"=w930) -> ("error out"=w929:errorcluster, "dup Message Queue"=w928:refnum<queue>)  [unwired: 7 in]
      }
      event "Exit": Value Change {
        n381 = event-data() -> ("CtlRef"=w932:refnum<vi>)  [unwired: 1 in]
        n382 = call "Enqueue Message.vi"("error in (no error)"=w938, "Message"="RT Exit", "Message Queue"=w936) -> ("error out"=w937:errorcluster, "dup Message Queue"=w935:refnum<queue>)  [unwired: 7 in]
        n383 = call "Enqueue Message.vi"("Priority Message? (F)"=TRUE, "error in (no error)"=w937, "Message"="Exit", "Message Queue"=w935) -> ("error out"=w942:errorcluster, "dup Message Queue"=w940:refnum<queue>)  [unwired: 6 in]
      }
      event "STOP DAQ": Value Change {
        n384 = event-data() -> ("CtlRef"=w943:refnum<vi>)  [unwired: 1 in]
        n385 = To Variant(anything=bool[] [FALSE, TRUE]) -> (Variant=w945:variant)
        n386 = call "Enqueue Message.vi"("error in (no error)"=w949, "Message Data"=w945, "Message"="Stop Daq", "Message Queue"=w950) -> ("error out"=w948:errorcluster, "dup Message Queue"=w947:refnum<queue>)  [unwired: 6 in]
      }
      event "Connect RT": Value Change {
        n387 = event-data() -> ("CtlRef"=w952:refnum<vi>)  [unwired: 1 in]
        n388 = call "Enqueue Message.vi"("error in (no error)"=w958, "Message"="Connect RT", "Message Queue"=w956) -> ("error out"=w957:errorcluster, "dup Message Queue"=w955:refnum<queue>)  [unwired: 7 in]
      }
      event User Event {
        n389 = event-data() -> ()  [unwired: 1 in, 2 out]
      }
      event "Connect ppsu": Value Change {
        n390 = event-data() -> ("CtlRef"=w962:refnum<vi>)  [unwired: 1 in]
        n391 = call "Enqueue Message.vi"("error in (no error)"=w965, "Message"="Connect PPSU", "Message Queue"=w968) -> ("error out"=w966:errorcluster, "dup Message Queue"=w967:refnum<queue>)  [unwired: 7 in]
      }
      event "DAQ SETTING": Value Change {
        n392 = event-data() -> ("CtlRef"=w969:refnum<vi>)  [unwired: 1 in]
        n393 = call "Enqueue Message.vi"("error in (no error)"=w975, "Message"="Daq Setting", "Message Queue"=w973) -> ("error out"=w974:errorcluster, "dup Message Queue"=w972:refnum<queue>)  [unwired: 7 in]
      }
      event "HOLD UPDATE": Value Change {
        n394 = event-data() -> ("CtlRef"=w976:refnum<vi>)  [unwired: 1 in]
        n395 = call "Enqueue Message.vi"("error in (no error)"=w981, "Message"="Hold Update", "Message Queue"=w982) -> ("error out"=w980:errorcluster, "dup Message Queue"=w979:refnum<queue>)  [unwired: 7 in]
      }
      event "STORAGE IP": Value Change {
        n396 = event-data() -> ("NewVal"=w986:string, "CtlRef"=w983:refnum<vi>)  [unwired: 1 in]
        n397 = To Variant(anything=w986) -> (Variant=w985:variant)
        n398 = call "Enqueue Message.vi"("error in (no error)"=w989, "Message Data"=w985, "Message"="Ip Config", "Message Queue"=w991) -> ("error out"=w988:errorcluster, "dup Message Queue"=w987:refnum<queue>)  [unwired: 6 in]
      }
      event "Log In Tool": Value Change {
        n399 = event-data() -> ("CtlRef"=w992:refnum<vi>)  [unwired: 1 in]
        n400 = call "Enqueue Message.vi"("error in (no error)"=w997, "Message"="Add User", "Message Queue"=w998) -> ("error out"=w996:errorcluster, "dup Message Queue"=w995:refnum<queue>)  [unwired: 7 in]
      }
      event "ABORT": Value Change {
        n401 = event-data() -> ("CtlRef"=w999:refnum<vi>)  [unwired: 1 in]
        n402 = call "Enqueue Message.vi"("error in (no error)"=w1004, "Message"="Abort", "Message Queue"=w1005) -> ("error out"=w1003:errorcluster, "dup Message Queue"=w1002:refnum<queue>)  [unwired: 7 in]
      }
      event "Connect Drive ATF": Value Change {
        n403 = event-data() -> ("CtlRef"=w1006:refnum<vi>)  [unwired: 1 in]
        n404 = call "Enqueue Message.vi"("error in (no error)"=w1012, "Message"="Connect Drive ATF", "Message Queue"=w1009) -> ("error out"=w1011:errorcluster, "dup Message Queue"=w1010:refnum<queue>)  [unwired: 7 in]
      }
      event "Alarm ack": Value Change {
        n405 = event-data() -> ("CtlRef"=w1013:refnum<vi>)  [unwired: 1 in]
        n406 = call "Enqueue Message.vi"("error in (no error)"=w1018, "Message"="Alarm Ack PPSU", "Message Queue"=w1016) -> ("error out"=w1017:errorcluster, "dup Message Queue"=w1015:refnum<queue>)  [unwired: 7 in]
      }
      event "Ms initialize": Value Change {
        n407 = event-data() -> ("CtlRef"=w1020:refnum<vi>)  [unwired: 1 in]
        n408 = call "Enqueue Message.vi"("error in (no error)"=w1026, "Message"="MS Initialize PPSU", "Message Queue"=w1023) -> ("error out"=w1025:errorcluster, "dup Message Queue"=w1024:refnum<queue>)  [unwired: 7 in]
      }
      event "update ppsu": Value Change {
        n409 = event-data() -> ("CtlRef"=w1027:refnum<vi>)  [unwired: 1 in]
        n410 = call "Enqueue Message.vi"("error in (no error)"=w1032, "Message"="Update PPSU Values", "Message Queue"=w1030) -> ("error out"=w1031:errorcluster, "dup Message Queue"=w1029:refnum<queue>)  [unwired: 7 in]
      }
      event "Exit Drive ATF": Value Change {
        n411 = event-data() -> ("CtlRef"=w1034:refnum<vi>)  [unwired: 1 in]
        n412 = call "Enqueue Message.vi"("error in (no error)"=w1040, "Message"="Exit Drive ATF", "Message Queue"=w1038) -> ("error out"=w1039:errorcluster, "dup Message Queue"=w1037:refnum<queue>)  [unwired: 7 in]
      }
      event "Update drive ATF": Value Change {
        n413 = event-data() -> ("CtlRef"=w1041:refnum<vi>)  [unwired: 1 in]
        n414 = call "Enqueue Message.vi"("error in (no error)"=w1047, "Message"="Update Drive ATF Values", "Message Queue"=w1045) -> ("error out"=w1046:errorcluster, "dup Message Queue"=w1044:refnum<queue>)  [unwired: 7 in]
      }
      event "STOP LOG": Value Change {
        n415 = event-data() -> ("CtlRef"=w1048:refnum<vi>)  [unwired: 1 in]
        n416 = call "Enqueue Message.vi"("error in (no error)"=w1053, "Message"="Stop Datalog", "Message Queue"=w1051) -> ("error out"=w1052:errorcluster, "dup Message Queue"=w1050:refnum<queue>)  [unwired: 7 in]
      }
      event "DC on": Value Change {
        n417 = event-data() -> ("CtlRef"=w1055:refnum<vi>)  [unwired: 1 in]
        n418 = call "Enqueue Message.vi"("error in (no error)"=w1061, "Message"="DC ON PPSU", "Message Queue"=w1059) -> ("error out"=w1060:errorcluster, "dup Message Queue"=w1058:refnum<queue>)  [unwired: 7 in]
      }
      event "DC off": Value Change {
        n419 = event-data() -> ("CtlRef"=w1062:refnum<vi>)  [unwired: 1 in]
        n420 = call "Enqueue Message.vi"("error in (no error)"=w1067, "Message"="DC OFF PPSU", "Message Queue"=w1064) -> ("error out"=w1066:errorcluster, "dup Message Queue"=w1065:refnum<queue>)  [unwired: 7 in]
      }
      event "Motor On ATF": Value Change {
        n421 = event-data() -> ("CtlRef"=w1069:refnum<vi>)  [unwired: 1 in]
        n422 = call "Enqueue Message.vi"("error in (no error)"=w1075, "Message"="Motor On ATF", "Message Queue"=w1073) -> ("error out"=w1074:errorcluster, "dup Message Queue"=w1072:refnum<queue>)  [unwired: 7 in]
      }
      event "Motor off ATF": Value Change {
        n423 = event-data() -> ("CtlRef"=w1076:refnum<vi>)  [unwired: 1 in]
        n424 = call "Enqueue Message.vi"("error in (no error)"=w1082, "Message"="Motor Off ATF", "Message Queue"=w1080) -> ("error out"=w1081:errorcluster, "dup Message Queue"=w1079:refnum<queue>)  [unwired: 7 in]
      }
      event "Gate driver ATF": Value Change {
        n425 = event-data() -> ("CtlRef"=w1083:refnum<vi>)  [unwired: 1 in]
        n426 = call "Enqueue Message.vi"("error in (no error)"=w1089, "Message"="Write DO", "Message Queue"=w1087) -> ("error out"=w1088:errorcluster, "dup Message Queue"=w1086:refnum<queue>)  [unwired: 7 in]
      }
      event "MCU reset ATF": Value Change {
        n427 = event-data() -> ("CtlRef"=w1090:refnum<vi>)  [unwired: 1 in]
        n428 = call "Enqueue Message.vi"("error in (no error)"=w1096, "Message"="Write DO", "Message Queue"=w1094) -> ("error out"=w1095:errorcluster, "dup Message Queue"=w1093:refnum<queue>)  [unwired: 7 in]
      }
      event "ADC reset ATF": Value Change {
        n429 = event-data() -> ("CtlRef"=w1097:refnum<vi>)  [unwired: 1 in]
        n430 = call "Enqueue Message.vi"("error in (no error)"=w1103, "Message"="Write DO", "Message Queue"=w1101) -> ("error out"=w1102:errorcluster, "dup Message Queue"=w1100:refnum<queue>)  [unwired: 7 in]
      }
      event "RT Stop": Value Change {
        n431 = event-data() -> ("CtlRef"=w1104:refnum<vi>)  [unwired: 1 in]
        n432 = call "Enqueue Message.vi"("error in (no error)"=w1110, "Message"="RT Stop", "Message Queue"=w1108) -> ("error out"=w1109:errorcluster, "dup Message Queue"=w1107:refnum<queue>)  [unwired: 7 in]
      }
      event "Enable/Disable IP": Value Change {
        n433 = event-data() -> ("CtlRef"=w1111:refnum<vi>)  [unwired: 1 in]
        n434 = call "Enqueue Message.vi"("error in (no error)"=w1116, "Message"="Ip Config", "Message Queue"=w1117) -> ("error out"=w1115:errorcluster, "dup Message Queue"=w1114:refnum<queue>)  [unwired: 7 in]
      }
    }
    n435 = case shown="No Error" w836 {
      selector: w836 -> [w848 _]
      tunnel: [w847 _] -> w834
      tunnel: w840 -> [_ w854]
      tunnel: w839 -> [w849 _]
      tunnel: [w849 FALSE] -> w838
      tunnel: w835 -> [w846 w851]
      tunnel: w832 -> [w845 w850]
      frame No Error {
        # "Event \nHandler"
        n436 = call "SeCrTs-Event Handler.vi"("error in (no error)"=w848, "Ev"=w845, "CtlRef"=w846) -> ("error out"=w847:errorcluster)  [unwired: 8 in]
      }
      frame Error {
        # "Event\nHandler"
        n437 = call "SeCrTs-Event Handler.vi"("Ev"=w850, "CtlRef"=w851) -> ()  [unwired: 9 in, 1 out]
        n438 = call "Enqueue Message.vi"("Priority Message? (F)"=TRUE, "Message"="Exit", "Message Queue"=w854) -> ()  [unwired: 7 in, 2 out]
      }
    }
    n439 = call "SeCrTs-Error handler P3.vi"("error in"=w834, "Message Queue"=w837) -> ("error out"=w833:errorcluster)  [unwired: 8 in, 1 out]
  }
  n440 = Unregister For Events(event registration refnum=w35, error in=w31) -> (error out=w34:errorcluster)
  n441 = call "Destroy User Event - Stop.vi"("error in (no error)"=w19, "User Event - Stop"=w24) -> ("error out"=w32:errorcluster)  [unwired: 9 in]
  n442 = Merge Errors(w34, w32, w19) -> (→"error out":errorcluster)
